vi "Userevent.vi"(0 "Timeout IN":i32, 7 "Source # startdelayLUT_coMD.vi?":bool, 9 "Source VI":string, 11 "Variable name":string, 12 "VI Match":bool, 13 "Value":variant) -> (4 "Timeout OUT":i32, 15 "shutdown?":bool)   [LabVIEW 2017]
uses:
  Custom Controls/display palette control.ctl
  Plugins/Macro Module/Macro Rule/subVIs/MacroRules_FGV_Commands.ctl
  CommonResource VIs/Timing/Timer Commands.ctl
  Custom Controls/pixel resolution enum.ctl
  Custom Controls/scan mode main settings tab.ctl
  Custom Controls/speed mode type def.ctl
  Custom Controls/experiment type.ctl
  Custom Controls/advanced settings inner tab CTL.ctl
  Custom Controls/MAIN Image panel tab Control type def.ctl
  Custom Controls/Histogram tab.ctl
  Custom Controls/trigger enum.ctl
  GFG/GFGDisplayRefsGet.vi
  GFG/GFGnumericGet.vi
  GFG/GFGfpRefGet.vi
  GFG/GFGbooleanGet.vi
  GFG/GFGImageRefsGet.vi
  GFG/GFG library.lvlib
panel:
  out "error out 6":errorcluster
  out "error out 5":errorcluster
  out "error out 4":errorcluster
  out "error out 3":errorcluster
  out "number of replacements":i32
  out "error out 2":errorcluster
  out "Source VI 2":string
  in  "String":string
  out "Maximum time delay observed":u32
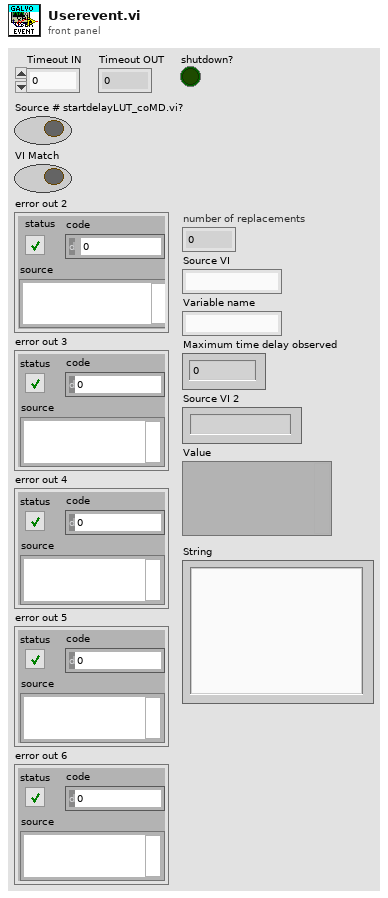
[diagram p1: front panel]
types:
  T1 = typedef "display palette control.ctl" = enum16{"standard", "high clipping red", "low clipping blue", "high and low clipping", "high / low (full range)"}
  T2 = typedef "MacroRules_FGV_Commands.ctl" = enum16{"Read File", "Get All", "Get Param and Flags"}
  T3 = typedef "Timer Commands.ctl" = enum16{"Clear All", "Start", "Pause", "Check Time"}
  T4 = enum8{"Enabled", "Disabled", "Disabled and Grayed Out"}
  T5 = typedef "pixel resolution enum.ctl" = enum16{"128 x 128", "256 x 128", "256 x 256", "512 x  64", "512 x 128", "512 x 256", "512 x 512", "1024 x 512", "1024 x 1024", "arbitrary"}
  T6 = typedef "scan mode main settings tab.ctl" = enum32{"2D frame", "2D line scan", "general settings", "Z Stack", "piezo"}
  T7 = typedef "experiment type.ctl" = string
  T8 = cluster{"xyvoltagefor2frames":dbl[][][], "x.pixels":dbl, "nomin.x.pixels":dbl, "y.pixels":dbl, "fill.fraction":dbl, "x.bidirectional":bool, "y.bidirectional":bool}
  T9 = enum32{"Page Enabled", "Page Disabled", "Page Disabled & Grayed"}
  T10 = typedef "advanced settings inner tab CTL.ctl" = enum32{"arb. frames", "AO", "AI", "channels", "trigger", "Zstack data"}
  T11 = typedef "MAIN Image panel tab Control type def.ctl" = enum32{"Channel 1", "Channel 2", "Channel 3", "Channel 4", "all channels", "RGB overlay", "ROI", "arbitrary line scan"}
  T12 = typedef "Histogram tab.ctl" = enum32{"hist Ch 1", "hist Ch 4", "hist Ch 3", "hist Ch 2"}
  T13 = typedef "trigger enum.ctl" = enum16{"legacy frame pulser PFI4", "continuous pulses", "single pulse", "trigger off"}
  T14 = cluster{"Channel 1 small":refnum<vi>, "Channel 2 small":refnum<vi>, "Channel 3 small":refnum<vi>, "Channel 4 small":refnum<vi>, "Channel 1 large":refnum<vi>, "Channel 2 large":refnum<vi>, "Channel 3 large":refnum<vi>, "Channel 4 large":refnum<vi>, "RGB overlay":refnum<vi>, "ROI Image display":refnum<vi>, "arb line scan display":refnum<vi>, "Channel 5 large":refnum<vi>}
  T15 = cluster{"WaveformChartRef":refnum<vi>, "DigitalRef":refnum<vi>, "ArrayRef":refnum<vi>, "TabControlRef":refnum<vi>, "EnumRef":refnum<vi>, "RingRef":refnum<vi>, "BooleanRef":refnum<vi>, "KnobRef":refnum<vi>, "SlideRef":refnum<vi>, "PathRef":refnum<vi>, "StringRef":refnum<vi>, "ComboBox":refnum<vi>, "WaveformGraphRef":refnum<vi>}
  T16 = typedef "IMAQ Image.ctl" = refnum<image>
  T17 = cluster{"Channel 1 small":T16, "Channel 2 small":T16, "Channel 3 small":T16, "Channel 4 small":T16, "Channel 1 large":T16, "Channel 2 large":T16, "Channel 3 large":T16, "Channel 4 large":T16, "RGB overlay":T16, "ROI Image display":T16, "arb line scan display":T16, "Channel 5 large":T16}
  T18 = typedef "speed mode type def.ctl" = u16
  T19 = typedef "LVStringsAndValuesArrayTypeDef.ctl" = cluster{"String":string, "Value":ext}[]
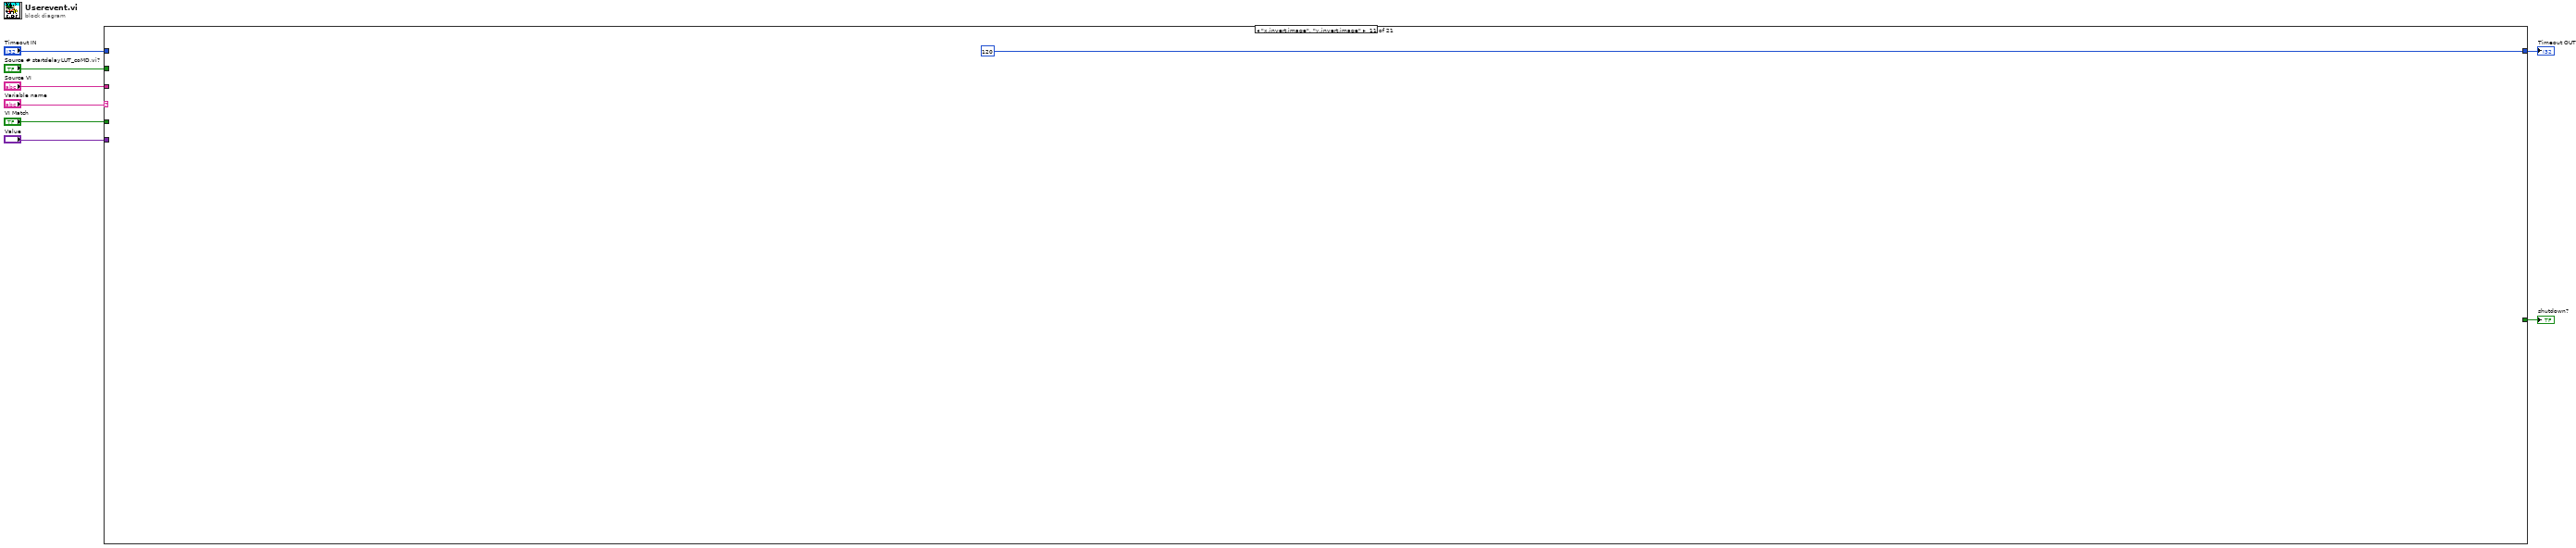
[diagram p0: block diagram]
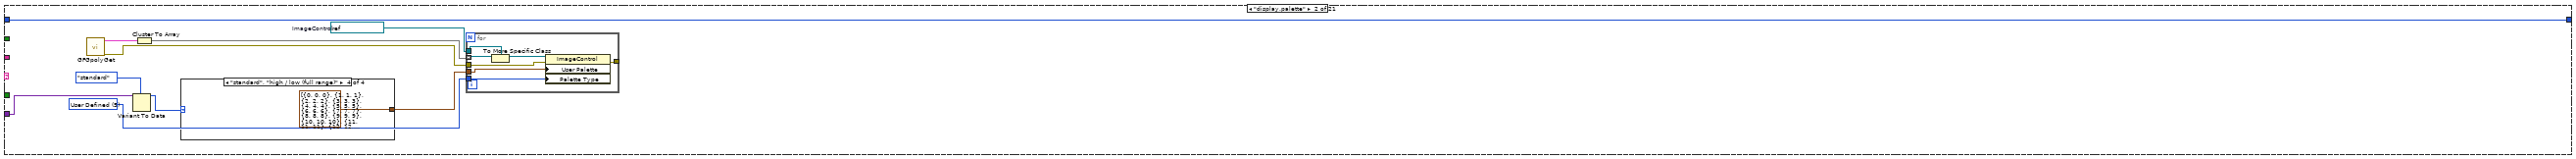
[diagram p3: hidden frame]
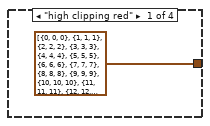
[diagram p4: hidden frame]
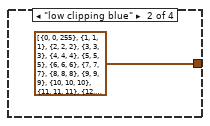
[diagram p5: hidden frame]
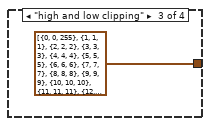
[diagram p6: hidden frame]
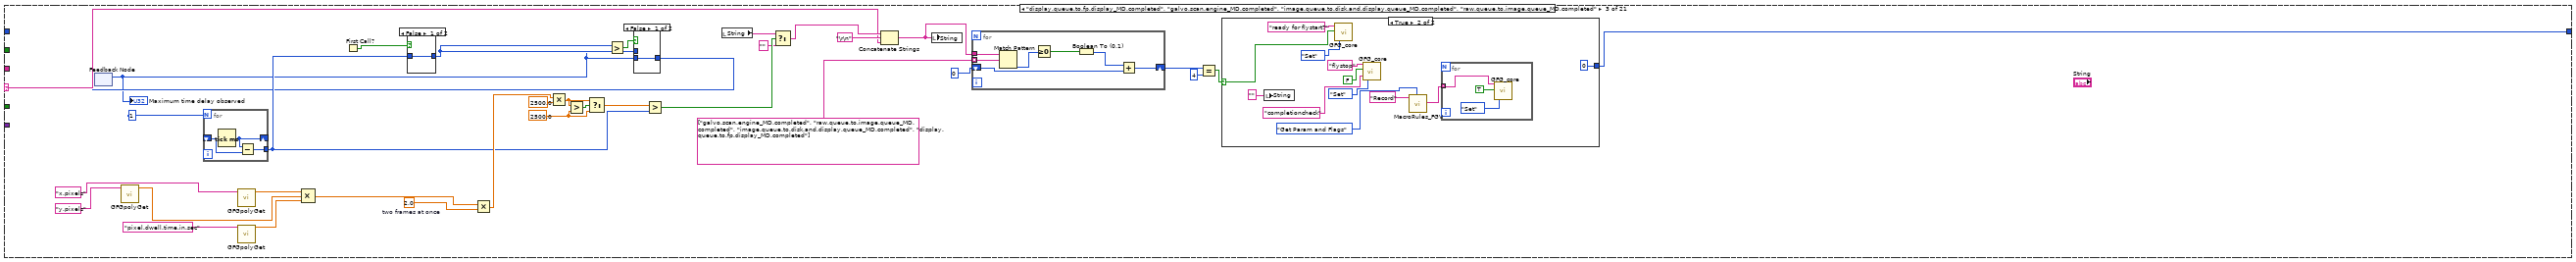
[diagram p7: hidden frame]
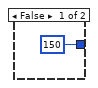
[diagram p8: hidden frame]
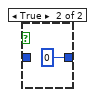
[diagram p9: hidden frame]
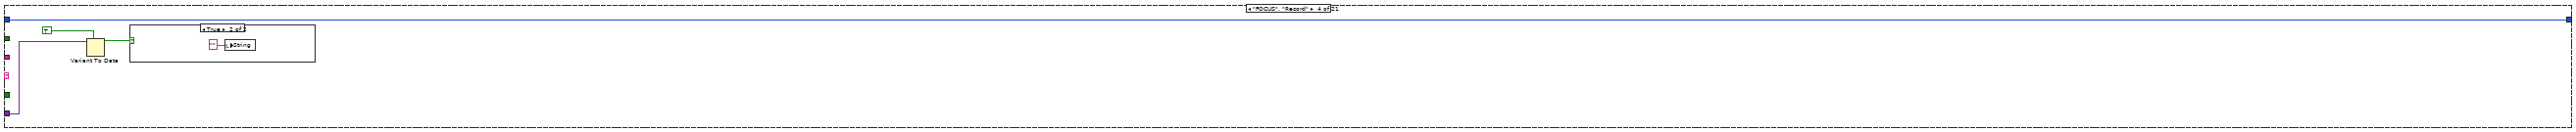
[diagram p11: hidden frame]
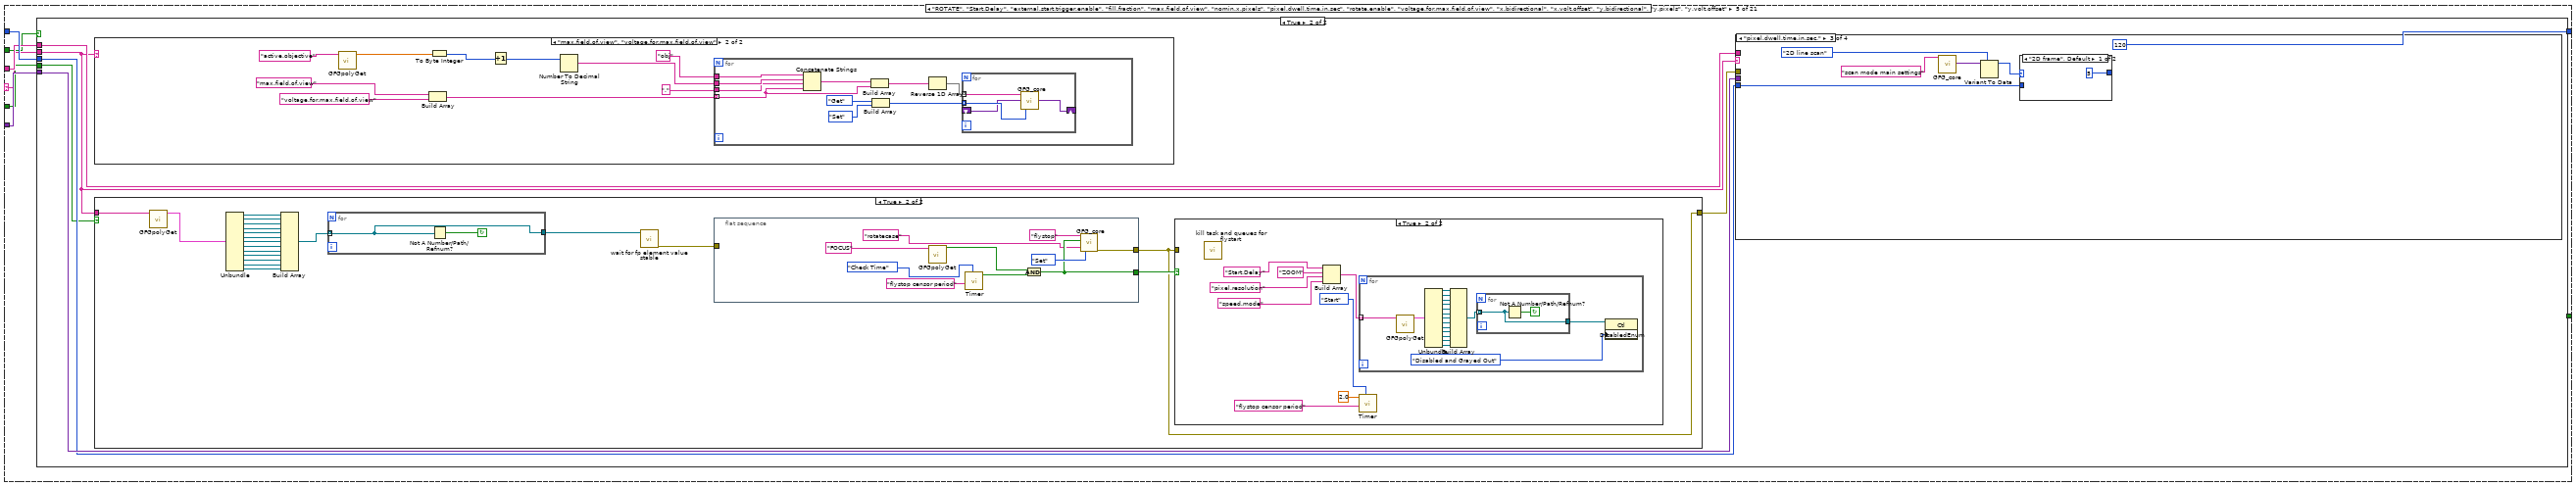
[diagram p13: hidden frame]
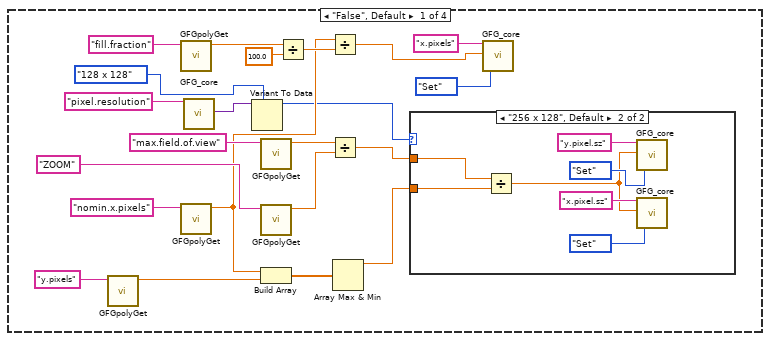
[diagram p18: hidden frame]
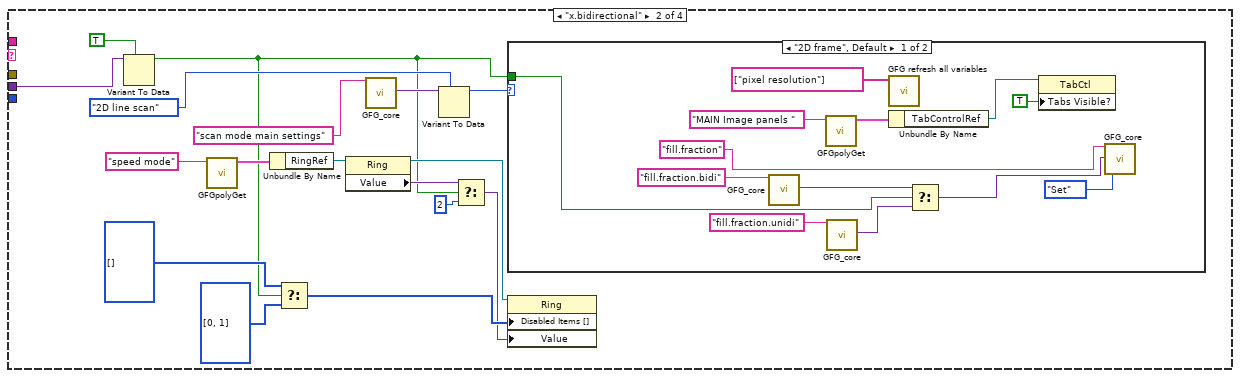
[diagram p20: hidden frame]
diagram:
  n1 = case shown="\"x.invert.image\", \"y.invert.image\"" "Variable name" {
    selector: "Variable name" -> [_ _ w54 _ w101 _ _ w311 _ w349 _ _ w620 _ _ _ _ _ _ _ _]
    tunnel: [_ _ _ _ _ _ _ _ _ _ _ _ _ _ _ _ _ _ TRUE _ _] -> w1
    tunnel: "Value" -> [_ w14 _ w98 w106 _ w289 _ _ w347 _ w601 w619 _ w712 w817 w872 w899 _ w953 w981]
    tunnel: [w9 w10 w53 w95 120 20 w302 w312 w338 w355 120 ("Timeout IN") w602 w618 w667 w708 w814 w871 w900 w919 w948 w975] -> w2
    tunnel: "Timeout IN" -> [w9 w10 _ w95 w105 _ w302 w312 w338 w344 _ w602 w618 w667 w709 w815 w871 w900 w919 w948 w975]
    tunnel: "Source VI" -> [_ _ _ _ w104 _ _ _ _ w353 _ _ _ w663 _ _ _ _ _ _ _]
    tunnel: "VI Match" -> [_ _ _ _ w102 _ _ _ _ w354 _ _ _ _ _ _ _ _ _ _ _]
    tunnel: "Source # startdelayLUT_coMD.vi?" -> [_ _ _ _ w100 _ _ _ _ _ _ _ _ _ _ _ _ _ _ _ _]
    frame "False", Default {
    }
    frame "display.palette" {
      w15 = u32 5 items=["Grayscale", "Binary", "Gradient", "Rainbow", "Temperature", "User Defined"] ("Palette:Palette Type")
      w17 = refnum<vi> refnum  # ImageControl
      n2 = call-poly "GFGpolyGet.vi"() -> ("error out"=w19:errorcluster, "DisplayRefsOut(generic class)"=w18:T14)  [unwired: 10 in]
      n3 = Variant To Data(type=display_palette_control."standard" ("display palette"), Variant=w14) -> (data=w12:T1)  [unwired: 1 in, 1 out]
      n4 = Cluster To Array(cluster=w18) -> (array=w16:refnum<vi>[])
      n5 = case shown="\"standard\", \"high / low (full range)\"" w12 {
        tunnel: [cluster{"Red":u8, "Green":u8, "Blue":u8}[] [{"Red"=0, "Green"=0, "Blue"=0}, {"Red"=1, "Green"=1, "Blue"=1}, {"Red"=2, "Green"=2, "Blue"=2}, {"Red"=3, "Green"=3, "Blue"=3}, {"Red"=4, "Green"=4, "Blue"=4}, {"Red"=5, "Green"=5, "Blue"=5}, {"Red"=6, "Green"=6, "Blue"=6}, {"Red"=7, "Green"=7, "Blue"=7}, {"Red"=8, "Green"=8, "Blue"=8}, {"Red"=9, "Green"=9, "Blue"=9}, {"Red"=10, "Green"=10, "Blue"=10}, {"Red"=11, "Green"=11, "Blue"=11}, {"Red"=12, "Green"=12, "Blue"=12}, {"Red"=13, "Green"=13, "Blue"=13}, {"Red"=14, "Green"=14, "Blue"=14}, {"Red"=15, "Green"=15, "Blue"=15}, {"Red"=16, "Green"=16, "Blue"=16}, {"Red"=17, "Green"=17, "Blue"=17}, {"Red"=18, "Green"=18, "Blue"=18}, {"Red"=19, "Green"=19, "Blue"=19}, {"Red"=20, "Green"=20, "Blue"=20}, {"Red"=21, "Green"=21, "Blue"=21}, {"Red"=22, "Green"=22, "Blue"=22}, {"Red"=23, "Green"=23, "Blue"=23}, {"Red"=24, "Green"=24, "Blue"=24}, {"Red"=25, "Green"=25, "Blue"=25}, {"Red"=26, "Green"=26, "Blue"=26}, {"Red"=27, "Green"=27, "Blue"=27}, {"Red"=28, "Green"=28, "Blue"=28}, {"Red"=29, "Green"=29, "Blue"=29}, {"Red"=30, "Green"=30, "Blue"=30}, {"Red"=31, "Green"=31, "Blue"=31}, {"Red"=32, "Green"=32, "Blue"=32}, {"Red"=33, "Green"=33, "Blue"=33}, {"Red"=34, "Green"=34, "Blue"=34}, {"Red"=35, "Green"=35, "Blue"=35}, {"Red"=36, "Green"=36, "Blue"=36}, {"Red"=37, "Green"=37, "Blue"=37}, {"Red"=38, "Green"=38, "Blue"=38}, {"Red"=39, "Green"=39, "Blue"=39}, {"Red"=40, "Green"=40, "Blue"=40}, {"Red"=41, "Green"=41, "Blue"=41}, {"Red"=42, "Green"=42, "Blue"=42}, {"Red"=43, "Green"=43, "Blue"=43}, {"Red"=44, "Green"=44, "Blue"=44}, {"Red"=45, "Green"=45, "Blue"=45}, {"Red"=46, "Green"=46, "Blue"=46}, {"Red"=47, "Green"=47, "Blue"=47}, {"Red"=48, "Green"=48, "Blue"=48}, {"Red"=49, "Green"=49, "Blue"=49}, {"Red"=50, "Green"=50, "Blue"=50}, {"Red"=51, "Green"=51, "Blue"=51}, {"Red"=52, "Green"=52, "Blue"=52}, {"Red"=53, "Green"=53, "Blue"=53}, {"Red"=54, "Green"=54, "Blue"=54}, {"Red"=55, "Green"=55, "Blue"=55}, {"Red"=56, "Green"=56, "Blue"=56}, {"Red"=57, "Green"=57, "Blue"=57}, {"Red"=58, "Green"=58, "Blue"=58}, {"Red"=59, "Green"=59, "Blue"=59}, {"Red"=60, "Green"=60, "Blue"=60}, {"Red"=61, "Green"=61, "Blue"=61}, {"Red"=62, "Green"=62, "Blue"=62}, {"Red"=63, "Green"=63, "Blue"=63}, {"Red"=64, "Green"=64, "Blue"=64}, {"Red"=65, "Green"=65, "Blue"=65}, {"Red"=66, "Green"=66, "Blue"=66}, {"Red"=67, "Green"=67, "Blue"=67}, {"Red"=68, "Green"=68, "Blue"=68}, {"Red"=69, "Green"=69, "Blue"=69}, {"Red"=70, "Green"=70, "Blue"=70}, {"Red"=71, "Green"=71, "Blue"=71}, {"Red"=72, "Green"=72, "Blue"=72}, {"Red"=73, "Green"=73, "Blue"=73}, {"Red"=74, "Green"=74, "Blue"=74}, {"Red"=75, "Green"=75, "Blue"=75}, {"Red"=76, "Green"=76, "Blue"=76}, {"Red"=77, "Green"=77, "Blue"=77}, {"Red"=78, "Green"=78, "Blue"=78}, {"Red"=79, "Green"=79, "Blue"=79}, {"Red"=80, "Green"=80, "Blue"=80}, {"Red"=81, "Green"=81, "Blue"=81}, {"Red"=82, "Green"=82, "Blue"=82}, {"Red"=83, "Green"=83, "Blue"=83}, {"Red"=84, "Green"=84, "Blue"=84}, {"Red"=85, "Green"=85, "Blue"=85}, {"Red"=86, "Green"=86, "Blue"=86}, {"Red"=87, "Green"=87, "Blue"=87}, {"Red"=88, "Green"=88, "Blue"=88}, {"Red"=89, "Green"=89, "Blue"=89}, {"Red"=90, "Green"=90, "Blue"=90}, {"Red"=91, "Green"=91, "Blue"=91}, {"Red"=92, "Green"=92, "Blue"=92}, {"Red"=93, "Green"=93, "Blue"=93}, {"Red"=94, "Green"=94, "Blue"=94}, {"Red"=95, "Green"=95, "Blue"=95}, {"Red"=96, "Green"=96, "Blue"=96}, {"Red"=97, "Green"=97, "Blue"=97}, {"Red"=98, "Green"=98, "Blue"=98}, {"Red"=99, "Green"=99, "Blue"=99}, {"Red"=100, "Green"=100, "Blue"=100}, {"Red"=101, "Green"=101, "Blue"=101}, {"Red"=102, "Green"=102, "Blue"=102}, {"Red"=103, "Green"=103, "Blue"=103}, {"Red"=104, "Green"=104, "Blue"=104}, {"Red"=105, "Green"=105, "Blue"=105}, {"Red"=106, "Green"=106, "Blue"=106}, {"Red"=107, "Green"=107, "Blue"=107}, {"Red"=108, "Green"=108, "Blue"=108}, {"Red"=109, "Green"=109, "Blue"=109}, {"Red"=110, "Green"=110, "Blue"=110}, {"Red"=111, "Green"=111, "Blue"=111}, {"Red"=112, "Green"=112, "Blue"=112}, {"Red"=113, "Green"=113, "Blue"=113}, {"Red"=114, "Green"=114, "Blue"=114}, {"Red"=115, "Green"=115, "Blue"=115}, {"Red"=116, "Green"=116, "Blue"=116}, {"Red"=117, "Green"=117, "Blue"=117}, {"Red"=118, "Green"=118, "Blue"=118}, {"Red"=119, "Green"=119, "Blue"=119}, {"Red"=120, "Green"=120, "Blue"=120}, {"Red"=121, "Green"=121, "Blue"=121}, {"Red"=122, "Green"=122, "Blue"=122}, {"Red"=123, "Green"=123, "Blue"=123}, {"Red"=124, "Green"=124, "Blue"=124}, {"Red"=125, "Green"=125, "Blue"=125}, {"Red"=126, "Green"=126, "Blue"=126}, {"Red"=127, "Green"=127, "Blue"=127}, {"Red"=128, "Green"=128, "Blue"=128}, {"Red"=129, "Green"=129, "Blue"=129}, {"Red"=130, "Green"=130, "Blue"=130}, {"Red"=131, "Green"=131, "Blue"=131}, {"Red"=132, "Green"=132, "Blue"=132}, {"Red"=133, "Green"=133, "Blue"=133}, {"Red"=134, "Green"=134, "Blue"=134}, {"Red"=135, "Green"=135, "Blue"=135}, {"Red"=136, "Green"=136, "Blue"=136}, {"Red"=137, "Green"=137, "Blue"=137}, {"Red"=138, "Green"=138, "Blue"=138}, {"Red"=139, "Green"=139, "Blue"=139}, {"Red"=140, "Green"=140, "Blue"=140}, {"Red"=141, "Green"=141, "Blue"=141}, {"Red"=142, "Green"=142, "Blue"=142}, {"Red"=143, "Green"=143, "Blue"=143}, {"Red"=144, "Green"=144, "Blue"=144}, {"Red"=145, "Green"=145, "Blue"=145}, {"Red"=146, "Green"=146, "Blue"=146}, {"Red"=147, "Green"=147, "Blue"=147}, {"Red"=148, "Green"=148, "Blue"=148}, {"Red"=149, "Green"=149, "Blue"=149}, {"Red"=150, "Green"=150, "Blue"=150}, {"Red"=151, "Green"=151, "Blue"=151}, {"Red"=152, "Green"=152, "Blue"=152}, {"Red"=153, "Green"=153, "Blue"=153}, {"Red"=154, "Green"=154, "Blue"=154}, {"Red"=155, "Green"=155, "Blue"=155}, {"Red"=156, "Green"=156, "Blue"=156}, {"Red"=157, "Green"=157, "Blue"=157}, {"Red"=158, "Green"=158, "Blue"=158}, {"Red"=159, "Green"=159, "Blue"=159}, {"Red"=160, "Green"=160, "Blue"=160}, {"Red"=161, "Green"=161, "Blue"=161}, {"Red"=162, "Green"=162, "Blue"=162}, {"Red"=163, "Green"=163, "Blue"=163}, {"Red"=164, "Green"=164, "Blue"=164}, {"Red"=165, "Green"=165, "Blue"=165}, {"Red"=166, "Green"=166, "Blue"=166}, {"Red"=167, "Green"=167, "Blue"=167}, {"Red"=168, "Green"=168, "Blue"=168}, {"Red"=169, "Green"=169, "Blue"=169}, {"Red"=170, "Green"=170, "Blue"=170}, {"Red"=171, "Green"=171, "Blue"=171}, {"Red"=172, "Green"=172, "Blue"=172}, {"Red"=173, "Green"=173, "Blue"=173}, {"Red"=174, "Green"=174, "Blue"=174}, {"Red"=175, "Green"=175, "Blue"=175}, {"Red"=176, "Green"=176, "Blue"=176}, {"Red"=177, "Green"=177, "Blue"=177}, {"Red"=178, "Green"=178, "Blue"=178}, {"Red"=179, "Green"=179, "Blue"=179}, {"Red"=180, "Green"=180, "Blue"=180}, {"Red"=181, "Green"=181, "Blue"=181}, {"Red"=182, "Green"=182, "Blue"=182}, {"Red"=183, "Green"=183, "Blue"=183}, {"Red"=184, "Green"=184, "Blue"=184}, {"Red"=185, "Green"=185, "Blue"=185}, {"Red"=186, "Green"=186, "Blue"=186}, {"Red"=187, "Green"=187, "Blue"=187}, {"Red"=188, "Green"=188, "Blue"=188}, {"Red"=189, "Green"=189, "Blue"=189}, {"Red"=190, "Green"=190, "Blue"=190}, {"Red"=191, "Green"=191, "Blue"=191}, {"Red"=192, "Green"=192, "Blue"=192}, {"Red"=193, "Green"=193, "Blue"=193}, {"Red"=194, "Green"=194, "Blue"=194}, {"Red"=195, "Green"=195, "Blue"=195}, {"Red"=196, "Green"=196, "Blue"=196}, {"Red"=197, "Green"=197, "Blue"=197}, {"Red"=198, "Green"=198, "Blue"=198}, {"Red"=199, "Green"=199, "Blue"=199}, {"Red"=200, "Green"=200, "Blue"=200}, {"Red"=201, "Green"=201, "Blue"=201}, {"Red"=202, "Green"=202, "Blue"=202}, {"Red"=203, "Green"=203, "Blue"=203}, {"Red"=204, "Green"=204, "Blue"=204}, {"Red"=205, "Green"=205, "Blue"=205}, {"Red"=206, "Green"=206, "Blue"=206}, {"Red"=207, "Green"=207, "Blue"=207}, {"Red"=208, "Green"=208, "Blue"=208}, {"Red"=209, "Green"=209, "Blue"=209}, {"Red"=210, "Green"=210, "Blue"=210}, {"Red"=211, "Green"=211, "Blue"=211}, {"Red"=212, "Green"=212, "Blue"=212}, {"Red"=213, "Green"=213, "Blue"=213}, {"Red"=214, "Green"=214, "Blue"=214}, {"Red"=215, "Green"=215, "Blue"=215}, {"Red"=216, "Green"=216, "Blue"=216}, {"Red"=217, "Green"=217, "Blue"=217}, {"Red"=218, "Green"=218, "Blue"=218}, {"Red"=219, "Green"=219, "Blue"=219}, {"Red"=220, "Green"=220, "Blue"=220}, {"Red"=221, "Green"=221, "Blue"=221}, {"Red"=222, "Green"=222, "Blue"=222}, {"Red"=223, "Green"=223, "Blue"=223}, {"Red"=224, "Green"=224, "Blue"=224}, {"Red"=225, "Green"=225, "Blue"=225}, {"Red"=226, "Green"=226, "Blue"=226}, {"Red"=227, "Green"=227, "Blue"=227}, {"Red"=228, "Green"=228, "Blue"=228}, {"Red"=229, "Green"=229, "Blue"=229}, {"Red"=230, "Green"=230, "Blue"=230}, {"Red"=231, "Green"=231, "Blue"=231}, {"Red"=232, "Green"=232, "Blue"=232}, {"Red"=233, "Green"=233, "Blue"=233}, {"Red"=234, "Green"=234, "Blue"=234}, {"Red"=235, "Green"=235, "Blue"=235}, {"Red"=236, "Green"=236, "Blue"=236}, {"Red"=237, "Green"=237, "Blue"=237}, {"Red"=238, "Green"=238, "Blue"=238}, {"Red"=239, "Green"=239, "Blue"=239}, {"Red"=240, "Green"=240, "Blue"=240}, {"Red"=241, "Green"=241, "Blue"=241}, {"Red"=242, "Green"=242, "Blue"=242}, {"Red"=243, "Green"=243, "Blue"=243}, {"Red"=244, "Green"=244, "Blue"=244}, {"Red"=245, "Green"=245, "Blue"=245}, {"Red"=246, "Green"=246, "Blue"=246}, {"Red"=247, "Green"=247, "Blue"=247}, {"Red"=248, "Green"=248, "Blue"=248}, {"Red"=249, "Green"=249, "Blue"=249}, {"Red"=250, "Green"=250, "Blue"=250}, {"Red"=251, "Green"=251, "Blue"=251}, {"Red"=252, "Green"=252, "Blue"=252}, {"Red"=253, "Green"=253, "Blue"=253}, {"Red"=254, "Green"=254, "Blue"=254}, {"Red"=255, "Green"=0, "Blue"=0}] ("Color Palette") cluster{"Red":u8, "Green":u8, "Blue":u8}[] [{"Red"=0, "Green"=0, "Blue"=255}, {"Red"=1, "Green"=1, "Blue"=1}, {"Red"=2, "Green"=2, "Blue"=2}, {"Red"=3, "Green"=3, "Blue"=3}, {"Red"=4, "Green"=4, "Blue"=4}, {"Red"=5, "Green"=5, "Blue"=5}, {"Red"=6, "Green"=6, "Blue"=6}, {"Red"=7, "Green"=7, "Blue"=7}, {"Red"=8, "Green"=8, "Blue"=8}, {"Red"=9, "Green"=9, "Blue"=9}, {"Red"=10, "Green"=10, "Blue"=10}, {"Red"=11, "Green"=11, "Blue"=11}, {"Red"=12, "Green"=12, "Blue"=12}, {"Red"=13, "Green"=13, "Blue"=13}, {"Red"=14, "Green"=14, "Blue"=14}, {"Red"=15, "Green"=15, "Blue"=15}, {"Red"=16, "Green"=16, "Blue"=16}, {"Red"=17, "Green"=17, "Blue"=17}, {"Red"=18, "Green"=18, "Blue"=18}, {"Red"=19, "Green"=19, "Blue"=19}, {"Red"=20, "Green"=20, "Blue"=20}, {"Red"=21, "Green"=21, "Blue"=21}, {"Red"=22, "Green"=22, "Blue"=22}, {"Red"=23, "Green"=23, "Blue"=23}, {"Red"=24, "Green"=24, "Blue"=24}, {"Red"=25, "Green"=25, "Blue"=25}, {"Red"=26, "Green"=26, "Blue"=26}, {"Red"=27, "Green"=27, "Blue"=27}, {"Red"=28, "Green"=28, "Blue"=28}, {"Red"=29, "Green"=29, "Blue"=29}, {"Red"=30, "Green"=30, "Blue"=30}, {"Red"=31, "Green"=31, "Blue"=31}, {"Red"=32, "Green"=32, "Blue"=32}, {"Red"=33, "Green"=33, "Blue"=33}, {"Red"=34, "Green"=34, "Blue"=34}, {"Red"=35, "Green"=35, "Blue"=35}, {"Red"=36, "Green"=36, "Blue"=36}, {"Red"=37, "Green"=37, "Blue"=37}, {"Red"=38, "Green"=38, "Blue"=38}, {"Red"=39, "Green"=39, "Blue"=39}, {"Red"=40, "Green"=40, "Blue"=40}, {"Red"=41, "Green"=41, "Blue"=41}, {"Red"=42, "Green"=42, "Blue"=42}, {"Red"=43, "Green"=43, "Blue"=43}, {"Red"=44, "Green"=44, "Blue"=44}, {"Red"=45, "Green"=45, "Blue"=45}, {"Red"=46, "Green"=46, "Blue"=46}, {"Red"=47, "Green"=47, "Blue"=47}, {"Red"=48, "Green"=48, "Blue"=48}, {"Red"=49, "Green"=49, "Blue"=49}, {"Red"=50, "Green"=50, "Blue"=50}, {"Red"=51, "Green"=51, "Blue"=51}, {"Red"=52, "Green"=52, "Blue"=52}, {"Red"=53, "Green"=53, "Blue"=53}, {"Red"=54, "Green"=54, "Blue"=54}, {"Red"=55, "Green"=55, "Blue"=55}, {"Red"=56, "Green"=56, "Blue"=56}, {"Red"=57, "Green"=57, "Blue"=57}, {"Red"=58, "Green"=58, "Blue"=58}, {"Red"=59, "Green"=59, "Blue"=59}, {"Red"=60, "Green"=60, "Blue"=60}, {"Red"=61, "Green"=61, "Blue"=61}, {"Red"=62, "Green"=62, "Blue"=62}, {"Red"=63, "Green"=63, "Blue"=63}, {"Red"=64, "Green"=64, "Blue"=64}, {"Red"=65, "Green"=65, "Blue"=65}, {"Red"=66, "Green"=66, "Blue"=66}, {"Red"=67, "Green"=67, "Blue"=67}, {"Red"=68, "Green"=68, "Blue"=68}, {"Red"=69, "Green"=69, "Blue"=69}, {"Red"=70, "Green"=70, "Blue"=70}, {"Red"=71, "Green"=71, "Blue"=71}, {"Red"=72, "Green"=72, "Blue"=72}, {"Red"=73, "Green"=73, "Blue"=73}, {"Red"=74, "Green"=74, "Blue"=74}, {"Red"=75, "Green"=75, "Blue"=75}, {"Red"=76, "Green"=76, "Blue"=76}, {"Red"=77, "Green"=77, "Blue"=77}, {"Red"=78, "Green"=78, "Blue"=78}, {"Red"=79, "Green"=79, "Blue"=79}, {"Red"=80, "Green"=80, "Blue"=80}, {"Red"=81, "Green"=81, "Blue"=81}, {"Red"=82, "Green"=82, "Blue"=82}, {"Red"=83, "Green"=83, "Blue"=83}, {"Red"=84, "Green"=84, "Blue"=84}, {"Red"=85, "Green"=85, "Blue"=85}, {"Red"=86, "Green"=86, "Blue"=86}, {"Red"=87, "Green"=87, "Blue"=87}, {"Red"=88, "Green"=88, "Blue"=88}, {"Red"=89, "Green"=89, "Blue"=89}, {"Red"=90, "Green"=90, "Blue"=90}, {"Red"=91, "Green"=91, "Blue"=91}, {"Red"=92, "Green"=92, "Blue"=92}, {"Red"=93, "Green"=93, "Blue"=93}, {"Red"=94, "Green"=94, "Blue"=94}, {"Red"=95, "Green"=95, "Blue"=95}, {"Red"=96, "Green"=96, "Blue"=96}, {"Red"=97, "Green"=97, "Blue"=97}, {"Red"=98, "Green"=98, "Blue"=98}, {"Red"=99, "Green"=99, "Blue"=99}, {"Red"=100, "Green"=100, "Blue"=100}, {"Red"=101, "Green"=101, "Blue"=101}, {"Red"=102, "Green"=102, "Blue"=102}, {"Red"=103, "Green"=103, "Blue"=103}, {"Red"=104, "Green"=104, "Blue"=104}, {"Red"=105, "Green"=105, "Blue"=105}, {"Red"=106, "Green"=106, "Blue"=106}, {"Red"=107, "Green"=107, "Blue"=107}, {"Red"=108, "Green"=108, "Blue"=108}, {"Red"=109, "Green"=109, "Blue"=109}, {"Red"=110, "Green"=110, "Blue"=110}, {"Red"=111, "Green"=111, "Blue"=111}, {"Red"=112, "Green"=112, "Blue"=112}, {"Red"=113, "Green"=113, "Blue"=113}, {"Red"=114, "Green"=114, "Blue"=114}, {"Red"=115, "Green"=115, "Blue"=115}, {"Red"=116, "Green"=116, "Blue"=116}, {"Red"=117, "Green"=117, "Blue"=117}, {"Red"=118, "Green"=118, "Blue"=118}, {"Red"=119, "Green"=119, "Blue"=119}, {"Red"=120, "Green"=120, "Blue"=120}, {"Red"=121, "Green"=121, "Blue"=121}, {"Red"=122, "Green"=122, "Blue"=122}, {"Red"=123, "Green"=123, "Blue"=123}, {"Red"=124, "Green"=124, "Blue"=124}, {"Red"=125, "Green"=125, "Blue"=125}, {"Red"=126, "Green"=126, "Blue"=126}, {"Red"=127, "Green"=127, "Blue"=127}, {"Red"=128, "Green"=128, "Blue"=128}, {"Red"=129, "Green"=129, "Blue"=129}, {"Red"=130, "Green"=130, "Blue"=130}, {"Red"=131, "Green"=131, "Blue"=131}, {"Red"=132, "Green"=132, "Blue"=132}, {"Red"=133, "Green"=133, "Blue"=133}, {"Red"=134, "Green"=134, "Blue"=134}, {"Red"=135, "Green"=135, "Blue"=135}, {"Red"=136, "Green"=136, "Blue"=136}, {"Red"=137, "Green"=137, "Blue"=137}, {"Red"=138, "Green"=138, "Blue"=138}, {"Red"=139, "Green"=139, "Blue"=139}, {"Red"=140, "Green"=140, "Blue"=140}, {"Red"=141, "Green"=141, "Blue"=141}, {"Red"=142, "Green"=142, "Blue"=142}, {"Red"=143, "Green"=143, "Blue"=143}, {"Red"=144, "Green"=144, "Blue"=144}, {"Red"=145, "Green"=145, "Blue"=145}, {"Red"=146, "Green"=146, "Blue"=146}, {"Red"=147, "Green"=147, "Blue"=147}, {"Red"=148, "Green"=148, "Blue"=148}, {"Red"=149, "Green"=149, "Blue"=149}, {"Red"=150, "Green"=150, "Blue"=150}, {"Red"=151, "Green"=151, "Blue"=151}, {"Red"=152, "Green"=152, "Blue"=152}, {"Red"=153, "Green"=153, "Blue"=153}, {"Red"=154, "Green"=154, "Blue"=154}, {"Red"=155, "Green"=155, "Blue"=155}, {"Red"=156, "Green"=156, "Blue"=156}, {"Red"=157, "Green"=157, "Blue"=157}, {"Red"=158, "Green"=158, "Blue"=158}, {"Red"=159, "Green"=159, "Blue"=159}, {"Red"=160, "Green"=160, "Blue"=160}, {"Red"=161, "Green"=161, "Blue"=161}, {"Red"=162, "Green"=162, "Blue"=162}, {"Red"=163, "Green"=163, "Blue"=163}, {"Red"=164, "Green"=164, "Blue"=164}, {"Red"=165, "Green"=165, "Blue"=165}, {"Red"=166, "Green"=166, "Blue"=166}, {"Red"=167, "Green"=167, "Blue"=167}, {"Red"=168, "Green"=168, "Blue"=168}, {"Red"=169, "Green"=169, "Blue"=169}, {"Red"=170, "Green"=170, "Blue"=170}, {"Red"=171, "Green"=171, "Blue"=171}, {"Red"=172, "Green"=172, "Blue"=172}, {"Red"=173, "Green"=173, "Blue"=173}, {"Red"=174, "Green"=174, "Blue"=174}, {"Red"=175, "Green"=175, "Blue"=175}, {"Red"=176, "Green"=176, "Blue"=176}, {"Red"=177, "Green"=177, "Blue"=177}, {"Red"=178, "Green"=178, "Blue"=178}, {"Red"=179, "Green"=179, "Blue"=179}, {"Red"=180, "Green"=180, "Blue"=180}, {"Red"=181, "Green"=181, "Blue"=181}, {"Red"=182, "Green"=182, "Blue"=182}, {"Red"=183, "Green"=183, "Blue"=183}, {"Red"=184, "Green"=184, "Blue"=184}, {"Red"=185, "Green"=185, "Blue"=185}, {"Red"=186, "Green"=186, "Blue"=186}, {"Red"=187, "Green"=187, "Blue"=187}, {"Red"=188, "Green"=188, "Blue"=188}, {"Red"=189, "Green"=189, "Blue"=189}, {"Red"=190, "Green"=190, "Blue"=190}, {"Red"=191, "Green"=191, "Blue"=191}, {"Red"=192, "Green"=192, "Blue"=192}, {"Red"=193, "Green"=193, "Blue"=193}, {"Red"=194, "Green"=194, "Blue"=194}, {"Red"=195, "Green"=195, "Blue"=195}, {"Red"=196, "Green"=196, "Blue"=196}, {"Red"=197, "Green"=197, "Blue"=197}, {"Red"=198, "Green"=198, "Blue"=198}, {"Red"=199, "Green"=199, "Blue"=199}, {"Red"=200, "Green"=200, "Blue"=200}, {"Red"=201, "Green"=201, "Blue"=201}, {"Red"=202, "Green"=202, "Blue"=202}, {"Red"=203, "Green"=203, "Blue"=203}, {"Red"=204, "Green"=204, "Blue"=204}, {"Red"=205, "Green"=205, "Blue"=205}, {"Red"=206, "Green"=206, "Blue"=206}, {"Red"=207, "Green"=207, "Blue"=207}, {"Red"=208, "Green"=208, "Blue"=208}, {"Red"=209, "Green"=209, "Blue"=209}, {"Red"=210, "Green"=210, "Blue"=210}, {"Red"=211, "Green"=211, "Blue"=211}, {"Red"=212, "Green"=212, "Blue"=212}, {"Red"=213, "Green"=213, "Blue"=213}, {"Red"=214, "Green"=214, "Blue"=214}, {"Red"=215, "Green"=215, "Blue"=215}, {"Red"=216, "Green"=216, "Blue"=216}, {"Red"=217, "Green"=217, "Blue"=217}, {"Red"=218, "Green"=218, "Blue"=218}, {"Red"=219, "Green"=219, "Blue"=219}, {"Red"=220, "Green"=220, "Blue"=220}, {"Red"=221, "Green"=221, "Blue"=221}, {"Red"=222, "Green"=222, "Blue"=222}, {"Red"=223, "Green"=223, "Blue"=223}, {"Red"=224, "Green"=224, "Blue"=224}, {"Red"=225, "Green"=225, "Blue"=225}, {"Red"=226, "Green"=226, "Blue"=226}, {"Red"=227, "Green"=227, "Blue"=227}, {"Red"=228, "Green"=228, "Blue"=228}, {"Red"=229, "Green"=229, "Blue"=229}, {"Red"=230, "Green"=230, "Blue"=230}, {"Red"=231, "Green"=231, "Blue"=231}, {"Red"=232, "Green"=232, "Blue"=232}, {"Red"=233, "Green"=233, "Blue"=233}, {"Red"=234, "Green"=234, "Blue"=234}, {"Red"=235, "Green"=235, "Blue"=235}, {"Red"=236, "Green"=236, "Blue"=236}, {"Red"=237, "Green"=237, "Blue"=237}, {"Red"=238, "Green"=238, "Blue"=238}, {"Red"=239, "Green"=239, "Blue"=239}, {"Red"=240, "Green"=240, "Blue"=240}, {"Red"=241, "Green"=241, "Blue"=241}, {"Red"=242, "Green"=242, "Blue"=242}, {"Red"=243, "Green"=243, "Blue"=243}, {"Red"=244, "Green"=244, "Blue"=244}, {"Red"=245, "Green"=245, "Blue"=245}, {"Red"=246, "Green"=246, "Blue"=246}, {"Red"=247, "Green"=247, "Blue"=247}, {"Red"=248, "Green"=248, "Blue"=248}, {"Red"=249, "Green"=249, "Blue"=249}, {"Red"=250, "Green"=250, "Blue"=250}, {"Red"=251, "Green"=251, "Blue"=251}, {"Red"=252, "Green"=252, "Blue"=252}, {"Red"=253, "Green"=253, "Blue"=253}, {"Red"=254, "Green"=254, "Blue"=254}, {"Red"=255, "Green"=255, "Blue"=255}] ("Color Palette") cluster{"Red":u8, "Green":u8, "Blue":u8}[] [{"Red"=0, "Green"=0, "Blue"=255}, {"Red"=1, "Green"=1, "Blue"=1}, {"Red"=2, "Green"=2, "Blue"=2}, {"Red"=3, "Green"=3, "Blue"=3}, {"Red"=4, "Green"=4, "Blue"=4}, {"Red"=5, "Green"=5, "Blue"=5}, {"Red"=6, "Green"=6, "Blue"=6}, {"Red"=7, "Green"=7, "Blue"=7}, {"Red"=8, "Green"=8, "Blue"=8}, {"Red"=9, "Green"=9, "Blue"=9}, {"Red"=10, "Green"=10, "Blue"=10}, {"Red"=11, "Green"=11, "Blue"=11}, {"Red"=12, "Green"=12, "Blue"=12}, {"Red"=13, "Green"=13, "Blue"=13}, {"Red"=14, "Green"=14, "Blue"=14}, {"Red"=15, "Green"=15, "Blue"=15}, {"Red"=16, "Green"=16, "Blue"=16}, {"Red"=17, "Green"=17, "Blue"=17}, {"Red"=18, "Green"=18, "Blue"=18}, {"Red"=19, "Green"=19, "Blue"=19}, {"Red"=20, "Green"=20, "Blue"=20}, {"Red"=21, "Green"=21, "Blue"=21}, {"Red"=22, "Green"=22, "Blue"=22}, {"Red"=23, "Green"=23, "Blue"=23}, {"Red"=24, "Green"=24, "Blue"=24}, {"Red"=25, "Green"=25, "Blue"=25}, {"Red"=26, "Green"=26, "Blue"=26}, {"Red"=27, "Green"=27, "Blue"=27}, {"Red"=28, "Green"=28, "Blue"=28}, {"Red"=29, "Green"=29, "Blue"=29}, {"Red"=30, "Green"=30, "Blue"=30}, {"Red"=31, "Green"=31, "Blue"=31}, {"Red"=32, "Green"=32, "Blue"=32}, {"Red"=33, "Green"=33, "Blue"=33}, {"Red"=34, "Green"=34, "Blue"=34}, {"Red"=35, "Green"=35, "Blue"=35}, {"Red"=36, "Green"=36, "Blue"=36}, {"Red"=37, "Green"=37, "Blue"=37}, {"Red"=38, "Green"=38, "Blue"=38}, {"Red"=39, "Green"=39, "Blue"=39}, {"Red"=40, "Green"=40, "Blue"=40}, {"Red"=41, "Green"=41, "Blue"=41}, {"Red"=42, "Green"=42, "Blue"=42}, {"Red"=43, "Green"=43, "Blue"=43}, {"Red"=44, "Green"=44, "Blue"=44}, {"Red"=45, "Green"=45, "Blue"=45}, {"Red"=46, "Green"=46, "Blue"=46}, {"Red"=47, "Green"=47, "Blue"=47}, {"Red"=48, "Green"=48, "Blue"=48}, {"Red"=49, "Green"=49, "Blue"=49}, {"Red"=50, "Green"=50, "Blue"=50}, {"Red"=51, "Green"=51, "Blue"=51}, {"Red"=52, "Green"=52, "Blue"=52}, {"Red"=53, "Green"=53, "Blue"=53}, {"Red"=54, "Green"=54, "Blue"=54}, {"Red"=55, "Green"=55, "Blue"=55}, {"Red"=56, "Green"=56, "Blue"=56}, {"Red"=57, "Green"=57, "Blue"=57}, {"Red"=58, "Green"=58, "Blue"=58}, {"Red"=59, "Green"=59, "Blue"=59}, {"Red"=60, "Green"=60, "Blue"=60}, {"Red"=61, "Green"=61, "Blue"=61}, {"Red"=62, "Green"=62, "Blue"=62}, {"Red"=63, "Green"=63, "Blue"=63}, {"Red"=64, "Green"=64, "Blue"=64}, {"Red"=65, "Green"=65, "Blue"=65}, {"Red"=66, "Green"=66, "Blue"=66}, {"Red"=67, "Green"=67, "Blue"=67}, {"Red"=68, "Green"=68, "Blue"=68}, {"Red"=69, "Green"=69, "Blue"=69}, {"Red"=70, "Green"=70, "Blue"=70}, {"Red"=71, "Green"=71, "Blue"=71}, {"Red"=72, "Green"=72, "Blue"=72}, {"Red"=73, "Green"=73, "Blue"=73}, {"Red"=74, "Green"=74, "Blue"=74}, {"Red"=75, "Green"=75, "Blue"=75}, {"Red"=76, "Green"=76, "Blue"=76}, {"Red"=77, "Green"=77, "Blue"=77}, {"Red"=78, "Green"=78, "Blue"=78}, {"Red"=79, "Green"=79, "Blue"=79}, {"Red"=80, "Green"=80, "Blue"=80}, {"Red"=81, "Green"=81, "Blue"=81}, {"Red"=82, "Green"=82, "Blue"=82}, {"Red"=83, "Green"=83, "Blue"=83}, {"Red"=84, "Green"=84, "Blue"=84}, {"Red"=85, "Green"=85, "Blue"=85}, {"Red"=86, "Green"=86, "Blue"=86}, {"Red"=87, "Green"=87, "Blue"=87}, {"Red"=88, "Green"=88, "Blue"=88}, {"Red"=89, "Green"=89, "Blue"=89}, {"Red"=90, "Green"=90, "Blue"=90}, {"Red"=91, "Green"=91, "Blue"=91}, {"Red"=92, "Green"=92, "Blue"=92}, {"Red"=93, "Green"=93, "Blue"=93}, {"Red"=94, "Green"=94, "Blue"=94}, {"Red"=95, "Green"=95, "Blue"=95}, {"Red"=96, "Green"=96, "Blue"=96}, {"Red"=97, "Green"=97, "Blue"=97}, {"Red"=98, "Green"=98, "Blue"=98}, {"Red"=99, "Green"=99, "Blue"=99}, {"Red"=100, "Green"=100, "Blue"=100}, {"Red"=101, "Green"=101, "Blue"=101}, {"Red"=102, "Green"=102, "Blue"=102}, {"Red"=103, "Green"=103, "Blue"=103}, {"Red"=104, "Green"=104, "Blue"=104}, {"Red"=105, "Green"=105, "Blue"=105}, {"Red"=106, "Green"=106, "Blue"=106}, {"Red"=107, "Green"=107, "Blue"=107}, {"Red"=108, "Green"=108, "Blue"=108}, {"Red"=109, "Green"=109, "Blue"=109}, {"Red"=110, "Green"=110, "Blue"=110}, {"Red"=111, "Green"=111, "Blue"=111}, {"Red"=112, "Green"=112, "Blue"=112}, {"Red"=113, "Green"=113, "Blue"=113}, {"Red"=114, "Green"=114, "Blue"=114}, {"Red"=115, "Green"=115, "Blue"=115}, {"Red"=116, "Green"=116, "Blue"=116}, {"Red"=117, "Green"=117, "Blue"=117}, {"Red"=118, "Green"=118, "Blue"=118}, {"Red"=119, "Green"=119, "Blue"=119}, {"Red"=120, "Green"=120, "Blue"=120}, {"Red"=121, "Green"=121, "Blue"=121}, {"Red"=122, "Green"=122, "Blue"=122}, {"Red"=123, "Green"=123, "Blue"=123}, {"Red"=124, "Green"=124, "Blue"=124}, {"Red"=125, "Green"=125, "Blue"=125}, {"Red"=126, "Green"=126, "Blue"=126}, {"Red"=127, "Green"=127, "Blue"=127}, {"Red"=128, "Green"=128, "Blue"=128}, {"Red"=129, "Green"=129, "Blue"=129}, {"Red"=130, "Green"=130, "Blue"=130}, {"Red"=131, "Green"=131, "Blue"=131}, {"Red"=132, "Green"=132, "Blue"=132}, {"Red"=133, "Green"=133, "Blue"=133}, {"Red"=134, "Green"=134, "Blue"=134}, {"Red"=135, "Green"=135, "Blue"=135}, {"Red"=136, "Green"=136, "Blue"=136}, {"Red"=137, "Green"=137, "Blue"=137}, {"Red"=138, "Green"=138, "Blue"=138}, {"Red"=139, "Green"=139, "Blue"=139}, {"Red"=140, "Green"=140, "Blue"=140}, {"Red"=141, "Green"=141, "Blue"=141}, {"Red"=142, "Green"=142, "Blue"=142}, {"Red"=143, "Green"=143, "Blue"=143}, {"Red"=144, "Green"=144, "Blue"=144}, {"Red"=145, "Green"=145, "Blue"=145}, {"Red"=146, "Green"=146, "Blue"=146}, {"Red"=147, "Green"=147, "Blue"=147}, {"Red"=148, "Green"=148, "Blue"=148}, {"Red"=149, "Green"=149, "Blue"=149}, {"Red"=150, "Green"=150, "Blue"=150}, {"Red"=151, "Green"=151, "Blue"=151}, {"Red"=152, "Green"=152, "Blue"=152}, {"Red"=153, "Green"=153, "Blue"=153}, {"Red"=154, "Green"=154, "Blue"=154}, {"Red"=155, "Green"=155, "Blue"=155}, {"Red"=156, "Green"=156, "Blue"=156}, {"Red"=157, "Green"=157, "Blue"=157}, {"Red"=158, "Green"=158, "Blue"=158}, {"Red"=159, "Green"=159, "Blue"=159}, {"Red"=160, "Green"=160, "Blue"=160}, {"Red"=161, "Green"=161, "Blue"=161}, {"Red"=162, "Green"=162, "Blue"=162}, {"Red"=163, "Green"=163, "Blue"=163}, {"Red"=164, "Green"=164, "Blue"=164}, {"Red"=165, "Green"=165, "Blue"=165}, {"Red"=166, "Green"=166, "Blue"=166}, {"Red"=167, "Green"=167, "Blue"=167}, {"Red"=168, "Green"=168, "Blue"=168}, {"Red"=169, "Green"=169, "Blue"=169}, {"Red"=170, "Green"=170, "Blue"=170}, {"Red"=171, "Green"=171, "Blue"=171}, {"Red"=172, "Green"=172, "Blue"=172}, {"Red"=173, "Green"=173, "Blue"=173}, {"Red"=174, "Green"=174, "Blue"=174}, {"Red"=175, "Green"=175, "Blue"=175}, {"Red"=176, "Green"=176, "Blue"=176}, {"Red"=177, "Green"=177, "Blue"=177}, {"Red"=178, "Green"=178, "Blue"=178}, {"Red"=179, "Green"=179, "Blue"=179}, {"Red"=180, "Green"=180, "Blue"=180}, {"Red"=181, "Green"=181, "Blue"=181}, {"Red"=182, "Green"=182, "Blue"=182}, {"Red"=183, "Green"=183, "Blue"=183}, {"Red"=184, "Green"=184, "Blue"=184}, {"Red"=185, "Green"=185, "Blue"=185}, {"Red"=186, "Green"=186, "Blue"=186}, {"Red"=187, "Green"=187, "Blue"=187}, {"Red"=188, "Green"=188, "Blue"=188}, {"Red"=189, "Green"=189, "Blue"=189}, {"Red"=190, "Green"=190, "Blue"=190}, {"Red"=191, "Green"=191, "Blue"=191}, {"Red"=192, "Green"=192, "Blue"=192}, {"Red"=193, "Green"=193, "Blue"=193}, {"Red"=194, "Green"=194, "Blue"=194}, {"Red"=195, "Green"=195, "Blue"=195}, {"Red"=196, "Green"=196, "Blue"=196}, {"Red"=197, "Green"=197, "Blue"=197}, {"Red"=198, "Green"=198, "Blue"=198}, {"Red"=199, "Green"=199, "Blue"=199}, {"Red"=200, "Green"=200, "Blue"=200}, {"Red"=201, "Green"=201, "Blue"=201}, {"Red"=202, "Green"=202, "Blue"=202}, {"Red"=203, "Green"=203, "Blue"=203}, {"Red"=204, "Green"=204, "Blue"=204}, {"Red"=205, "Green"=205, "Blue"=205}, {"Red"=206, "Green"=206, "Blue"=206}, {"Red"=207, "Green"=207, "Blue"=207}, {"Red"=208, "Green"=208, "Blue"=208}, {"Red"=209, "Green"=209, "Blue"=209}, {"Red"=210, "Green"=210, "Blue"=210}, {"Red"=211, "Green"=211, "Blue"=211}, {"Red"=212, "Green"=212, "Blue"=212}, {"Red"=213, "Green"=213, "Blue"=213}, {"Red"=214, "Green"=214, "Blue"=214}, {"Red"=215, "Green"=215, "Blue"=215}, {"Red"=216, "Green"=216, "Blue"=216}, {"Red"=217, "Green"=217, "Blue"=217}, {"Red"=218, "Green"=218, "Blue"=218}, {"Red"=219, "Green"=219, "Blue"=219}, {"Red"=220, "Green"=220, "Blue"=220}, {"Red"=221, "Green"=221, "Blue"=221}, {"Red"=222, "Green"=222, "Blue"=222}, {"Red"=223, "Green"=223, "Blue"=223}, {"Red"=224, "Green"=224, "Blue"=224}, {"Red"=225, "Green"=225, "Blue"=225}, {"Red"=226, "Green"=226, "Blue"=226}, {"Red"=227, "Green"=227, "Blue"=227}, {"Red"=228, "Green"=228, "Blue"=228}, {"Red"=229, "Green"=229, "Blue"=229}, {"Red"=230, "Green"=230, "Blue"=230}, {"Red"=231, "Green"=231, "Blue"=231}, {"Red"=232, "Green"=232, "Blue"=232}, {"Red"=233, "Green"=233, "Blue"=233}, {"Red"=234, "Green"=234, "Blue"=234}, {"Red"=235, "Green"=235, "Blue"=235}, {"Red"=236, "Green"=236, "Blue"=236}, {"Red"=237, "Green"=237, "Blue"=237}, {"Red"=238, "Green"=238, "Blue"=238}, {"Red"=239, "Green"=239, "Blue"=239}, {"Red"=240, "Green"=240, "Blue"=240}, {"Red"=241, "Green"=241, "Blue"=241}, {"Red"=242, "Green"=242, "Blue"=242}, {"Red"=243, "Green"=243, "Blue"=243}, {"Red"=244, "Green"=244, "Blue"=244}, {"Red"=245, "Green"=245, "Blue"=245}, {"Red"=246, "Green"=246, "Blue"=246}, {"Red"=247, "Green"=247, "Blue"=247}, {"Red"=248, "Green"=248, "Blue"=248}, {"Red"=249, "Green"=249, "Blue"=249}, {"Red"=250, "Green"=250, "Blue"=250}, {"Red"=251, "Green"=251, "Blue"=251}, {"Red"=252, "Green"=252, "Blue"=252}, {"Red"=253, "Green"=253, "Blue"=253}, {"Red"=254, "Green"=254, "Blue"=254}, {"Red"=255, "Green"=0, "Blue"=0}] ("Color Palette") cluster{"Red":u8, "Green":u8, "Blue":u8}[] [{"Red"=0, "Green"=0, "Blue"=0}, {"Red"=1, "Green"=1, "Blue"=1}, {"Red"=2, "Green"=2, "Blue"=2}, {"Red"=3, "Green"=3, "Blue"=3}, {"Red"=4, "Green"=4, "Blue"=4}, {"Red"=5, "Green"=5, "Blue"=5}, {"Red"=6, "Green"=6, "Blue"=6}, {"Red"=7, "Green"=7, "Blue"=7}, {"Red"=8, "Green"=8, "Blue"=8}, {"Red"=9, "Green"=9, "Blue"=9}, {"Red"=10, "Green"=10, "Blue"=10}, {"Red"=11, "Green"=11, "Blue"=11}, {"Red"=12, "Green"=12, "Blue"=12}, {"Red"=13, "Green"=13, "Blue"=13}, {"Red"=14, "Green"=14, "Blue"=14}, {"Red"=15, "Green"=15, "Blue"=15}, {"Red"=16, "Green"=16, "Blue"=16}, {"Red"=17, "Green"=17, "Blue"=17}, {"Red"=18, "Green"=18, "Blue"=18}, {"Red"=19, "Green"=19, "Blue"=19}, {"Red"=20, "Green"=20, "Blue"=20}, {"Red"=21, "Green"=21, "Blue"=21}, {"Red"=22, "Green"=22, "Blue"=22}, {"Red"=23, "Green"=23, "Blue"=23}, {"Red"=24, "Green"=24, "Blue"=24}, {"Red"=25, "Green"=25, "Blue"=25}, {"Red"=26, "Green"=26, "Blue"=26}, {"Red"=27, "Green"=27, "Blue"=27}, {"Red"=28, "Green"=28, "Blue"=28}, {"Red"=29, "Green"=29, "Blue"=29}, {"Red"=30, "Green"=30, "Blue"=30}, {"Red"=31, "Green"=31, "Blue"=31}, {"Red"=32, "Green"=32, "Blue"=32}, {"Red"=33, "Green"=33, "Blue"=33}, {"Red"=34, "Green"=34, "Blue"=34}, {"Red"=35, "Green"=35, "Blue"=35}, {"Red"=36, "Green"=36, "Blue"=36}, {"Red"=37, "Green"=37, "Blue"=37}, {"Red"=38, "Green"=38, "Blue"=38}, {"Red"=39, "Green"=39, "Blue"=39}, {"Red"=40, "Green"=40, "Blue"=40}, {"Red"=41, "Green"=41, "Blue"=41}, {"Red"=42, "Green"=42, "Blue"=42}, {"Red"=43, "Green"=43, "Blue"=43}, {"Red"=44, "Green"=44, "Blue"=44}, {"Red"=45, "Green"=45, "Blue"=45}, {"Red"=46, "Green"=46, "Blue"=46}, {"Red"=47, "Green"=47, "Blue"=47}, {"Red"=48, "Green"=48, "Blue"=48}, {"Red"=49, "Green"=49, "Blue"=49}, {"Red"=50, "Green"=50, "Blue"=50}, {"Red"=51, "Green"=51, "Blue"=51}, {"Red"=52, "Green"=52, "Blue"=52}, {"Red"=53, "Green"=53, "Blue"=53}, {"Red"=54, "Green"=54, "Blue"=54}, {"Red"=55, "Green"=55, "Blue"=55}, {"Red"=56, "Green"=56, "Blue"=56}, {"Red"=57, "Green"=57, "Blue"=57}, {"Red"=58, "Green"=58, "Blue"=58}, {"Red"=59, "Green"=59, "Blue"=59}, {"Red"=60, "Green"=60, "Blue"=60}, {"Red"=61, "Green"=61, "Blue"=61}, {"Red"=62, "Green"=62, "Blue"=62}, {"Red"=63, "Green"=63, "Blue"=63}, {"Red"=64, "Green"=64, "Blue"=64}, {"Red"=65, "Green"=65, "Blue"=65}, {"Red"=66, "Green"=66, "Blue"=66}, {"Red"=67, "Green"=67, "Blue"=67}, {"Red"=68, "Green"=68, "Blue"=68}, {"Red"=69, "Green"=69, "Blue"=69}, {"Red"=70, "Green"=70, "Blue"=70}, {"Red"=71, "Green"=71, "Blue"=71}, {"Red"=72, "Green"=72, "Blue"=72}, {"Red"=73, "Green"=73, "Blue"=73}, {"Red"=74, "Green"=74, "Blue"=74}, {"Red"=75, "Green"=75, "Blue"=75}, {"Red"=76, "Green"=76, "Blue"=76}, {"Red"=77, "Green"=77, "Blue"=77}, {"Red"=78, "Green"=78, "Blue"=78}, {"Red"=79, "Green"=79, "Blue"=79}, {"Red"=80, "Green"=80, "Blue"=80}, {"Red"=81, "Green"=81, "Blue"=81}, {"Red"=82, "Green"=82, "Blue"=82}, {"Red"=83, "Green"=83, "Blue"=83}, {"Red"=84, "Green"=84, "Blue"=84}, {"Red"=85, "Green"=85, "Blue"=85}, {"Red"=86, "Green"=86, "Blue"=86}, {"Red"=87, "Green"=87, "Blue"=87}, {"Red"=88, "Green"=88, "Blue"=88}, {"Red"=89, "Green"=89, "Blue"=89}, {"Red"=90, "Green"=90, "Blue"=90}, {"Red"=91, "Green"=91, "Blue"=91}, {"Red"=92, "Green"=92, "Blue"=92}, {"Red"=93, "Green"=93, "Blue"=93}, {"Red"=94, "Green"=94, "Blue"=94}, {"Red"=95, "Green"=95, "Blue"=95}, {"Red"=96, "Green"=96, "Blue"=96}, {"Red"=97, "Green"=97, "Blue"=97}, {"Red"=98, "Green"=98, "Blue"=98}, {"Red"=99, "Green"=99, "Blue"=99}, {"Red"=100, "Green"=100, "Blue"=100}, {"Red"=101, "Green"=101, "Blue"=101}, {"Red"=102, "Green"=102, "Blue"=102}, {"Red"=103, "Green"=103, "Blue"=103}, {"Red"=104, "Green"=104, "Blue"=104}, {"Red"=105, "Green"=105, "Blue"=105}, {"Red"=106, "Green"=106, "Blue"=106}, {"Red"=107, "Green"=107, "Blue"=107}, {"Red"=108, "Green"=108, "Blue"=108}, {"Red"=109, "Green"=109, "Blue"=109}, {"Red"=110, "Green"=110, "Blue"=110}, {"Red"=111, "Green"=111, "Blue"=111}, {"Red"=112, "Green"=112, "Blue"=112}, {"Red"=113, "Green"=113, "Blue"=113}, {"Red"=114, "Green"=114, "Blue"=114}, {"Red"=115, "Green"=115, "Blue"=115}, {"Red"=116, "Green"=116, "Blue"=116}, {"Red"=117, "Green"=117, "Blue"=117}, {"Red"=118, "Green"=118, "Blue"=118}, {"Red"=119, "Green"=119, "Blue"=119}, {"Red"=120, "Green"=120, "Blue"=120}, {"Red"=121, "Green"=121, "Blue"=121}, {"Red"=122, "Green"=122, "Blue"=122}, {"Red"=123, "Green"=123, "Blue"=123}, {"Red"=124, "Green"=124, "Blue"=124}, {"Red"=125, "Green"=125, "Blue"=125}, {"Red"=126, "Green"=126, "Blue"=126}, {"Red"=127, "Green"=127, "Blue"=127}, {"Red"=128, "Green"=128, "Blue"=128}, {"Red"=129, "Green"=129, "Blue"=129}, {"Red"=130, "Green"=130, "Blue"=130}, {"Red"=131, "Green"=131, "Blue"=131}, {"Red"=132, "Green"=132, "Blue"=132}, {"Red"=133, "Green"=133, "Blue"=133}, {"Red"=134, "Green"=134, "Blue"=134}, {"Red"=135, "Green"=135, "Blue"=135}, {"Red"=136, "Green"=136, "Blue"=136}, {"Red"=137, "Green"=137, "Blue"=137}, {"Red"=138, "Green"=138, "Blue"=138}, {"Red"=139, "Green"=139, "Blue"=139}, {"Red"=140, "Green"=140, "Blue"=140}, {"Red"=141, "Green"=141, "Blue"=141}, {"Red"=142, "Green"=142, "Blue"=142}, {"Red"=143, "Green"=143, "Blue"=143}, {"Red"=144, "Green"=144, "Blue"=144}, {"Red"=145, "Green"=145, "Blue"=145}, {"Red"=146, "Green"=146, "Blue"=146}, {"Red"=147, "Green"=147, "Blue"=147}, {"Red"=148, "Green"=148, "Blue"=148}, {"Red"=149, "Green"=149, "Blue"=149}, {"Red"=150, "Green"=150, "Blue"=150}, {"Red"=151, "Green"=151, "Blue"=151}, {"Red"=152, "Green"=152, "Blue"=152}, {"Red"=153, "Green"=153, "Blue"=153}, {"Red"=154, "Green"=154, "Blue"=154}, {"Red"=155, "Green"=155, "Blue"=155}, {"Red"=156, "Green"=156, "Blue"=156}, {"Red"=157, "Green"=157, "Blue"=157}, {"Red"=158, "Green"=158, "Blue"=158}, {"Red"=159, "Green"=159, "Blue"=159}, {"Red"=160, "Green"=160, "Blue"=160}, {"Red"=161, "Green"=161, "Blue"=161}, {"Red"=162, "Green"=162, "Blue"=162}, {"Red"=163, "Green"=163, "Blue"=163}, {"Red"=164, "Green"=164, "Blue"=164}, {"Red"=165, "Green"=165, "Blue"=165}, {"Red"=166, "Green"=166, "Blue"=166}, {"Red"=167, "Green"=167, "Blue"=167}, {"Red"=168, "Green"=168, "Blue"=168}, {"Red"=169, "Green"=169, "Blue"=169}, {"Red"=170, "Green"=170, "Blue"=170}, {"Red"=171, "Green"=171, "Blue"=171}, {"Red"=172, "Green"=172, "Blue"=172}, {"Red"=173, "Green"=173, "Blue"=173}, {"Red"=174, "Green"=174, "Blue"=174}, {"Red"=175, "Green"=175, "Blue"=175}, {"Red"=176, "Green"=176, "Blue"=176}, {"Red"=177, "Green"=177, "Blue"=177}, {"Red"=178, "Green"=178, "Blue"=178}, {"Red"=179, "Green"=179, "Blue"=179}, {"Red"=180, "Green"=180, "Blue"=180}, {"Red"=181, "Green"=181, "Blue"=181}, {"Red"=182, "Green"=182, "Blue"=182}, {"Red"=183, "Green"=183, "Blue"=183}, {"Red"=184, "Green"=184, "Blue"=184}, {"Red"=185, "Green"=185, "Blue"=185}, {"Red"=186, "Green"=186, "Blue"=186}, {"Red"=187, "Green"=187, "Blue"=187}, {"Red"=188, "Green"=188, "Blue"=188}, {"Red"=189, "Green"=189, "Blue"=189}, {"Red"=190, "Green"=190, "Blue"=190}, {"Red"=191, "Green"=191, "Blue"=191}, {"Red"=192, "Green"=192, "Blue"=192}, {"Red"=193, "Green"=193, "Blue"=193}, {"Red"=194, "Green"=194, "Blue"=194}, {"Red"=195, "Green"=195, "Blue"=195}, {"Red"=196, "Green"=196, "Blue"=196}, {"Red"=197, "Green"=197, "Blue"=197}, {"Red"=198, "Green"=198, "Blue"=198}, {"Red"=199, "Green"=199, "Blue"=199}, {"Red"=200, "Green"=200, "Blue"=200}, {"Red"=201, "Green"=201, "Blue"=201}, {"Red"=202, "Green"=202, "Blue"=202}, {"Red"=203, "Green"=203, "Blue"=203}, {"Red"=204, "Green"=204, "Blue"=204}, {"Red"=205, "Green"=205, "Blue"=205}, {"Red"=206, "Green"=206, "Blue"=206}, {"Red"=207, "Green"=207, "Blue"=207}, {"Red"=208, "Green"=208, "Blue"=208}, {"Red"=209, "Green"=209, "Blue"=209}, {"Red"=210, "Green"=210, "Blue"=210}, {"Red"=211, "Green"=211, "Blue"=211}, {"Red"=212, "Green"=212, "Blue"=212}, {"Red"=213, "Green"=213, "Blue"=213}, {"Red"=214, "Green"=214, "Blue"=214}, {"Red"=215, "Green"=215, "Blue"=215}, {"Red"=216, "Green"=216, "Blue"=216}, {"Red"=217, "Green"=217, "Blue"=217}, {"Red"=218, "Green"=218, "Blue"=218}, {"Red"=219, "Green"=219, "Blue"=219}, {"Red"=220, "Green"=220, "Blue"=220}, {"Red"=221, "Green"=221, "Blue"=221}, {"Red"=222, "Green"=222, "Blue"=222}, {"Red"=223, "Green"=223, "Blue"=223}, {"Red"=224, "Green"=224, "Blue"=224}, {"Red"=225, "Green"=225, "Blue"=225}, {"Red"=226, "Green"=226, "Blue"=226}, {"Red"=227, "Green"=227, "Blue"=227}, {"Red"=228, "Green"=228, "Blue"=228}, {"Red"=229, "Green"=229, "Blue"=229}, {"Red"=230, "Green"=230, "Blue"=230}, {"Red"=231, "Green"=231, "Blue"=231}, {"Red"=232, "Green"=232, "Blue"=232}, {"Red"=233, "Green"=233, "Blue"=233}, {"Red"=234, "Green"=234, "Blue"=234}, {"Red"=235, "Green"=235, "Blue"=235}, {"Red"=236, "Green"=236, "Blue"=236}, {"Red"=237, "Green"=237, "Blue"=237}, {"Red"=238, "Green"=238, "Blue"=238}, {"Red"=239, "Green"=239, "Blue"=239}, {"Red"=240, "Green"=240, "Blue"=240}, {"Red"=241, "Green"=241, "Blue"=241}, {"Red"=242, "Green"=242, "Blue"=242}, {"Red"=243, "Green"=243, "Blue"=243}, {"Red"=244, "Green"=244, "Blue"=244}, {"Red"=245, "Green"=245, "Blue"=245}, {"Red"=246, "Green"=246, "Blue"=246}, {"Red"=247, "Green"=247, "Blue"=247}, {"Red"=248, "Green"=248, "Blue"=248}, {"Red"=249, "Green"=249, "Blue"=249}, {"Red"=250, "Green"=250, "Blue"=250}, {"Red"=251, "Green"=251, "Blue"=251}, {"Red"=252, "Green"=252, "Blue"=252}, {"Red"=253, "Green"=253, "Blue"=253}, {"Red"=254, "Green"=254, "Blue"=254}, {"Red"=255, "Green"=255, "Blue"=255}] ("Color Palette")] -> w11
        frame "high clipping red" {
        }
        frame "low clipping blue" {
        }
        frame "high and low clipping" {
        }
        frame "standard", "high / low (full range)" {
        }
      }
      n6 = for {
        tunnel: w16 -> [w30] mode=indexing
        tunnel: w11 -> [w24]
        tunnel: w15 -> [w25]
        tunnel: w19 -> [w26]
        tunnel: [w27] -> _
        tunnel: w17 -> [w29]
        n7 = To More Specific Class(target class=w29, reference=w30) -> (specific class reference=w28:refnum<vi>)  [unwired: 1 in, 1 out]
        n8 = property class="ImageControl"(reference=w28, error in=w26, "User Palette"=w24, "Palette Type"=w25) -> (error out=w27:errorcluster)  [unwired: 1 out]
      }
    }
    frame "display.queue.to.fp.display_MD.completed", "galvo.scan.engine_MD.completed", "image.queue.to.disk.and.display.queue_MD.completed", "raw.queue.to.image.queue_MD.completed" {
      w34 = 2500.0 ("y")
      w52 = 2.0  # two frames at once
      n9 = feedback #1() -> (w37:u32)  [unwired: 1 in]
      "Maximum time delay observed" <- w37
      n10 = call-poly "GFGpolyGet.vi"("Variable Name in"="y.pixels") -> ("Numeric"=w45:dbl)  [unwired: 8 in, 2 out]
      n11 = for {
        N: 1 -> [_]
        shift-right: [w85] -> _
        shift-left: _ -> [w87]
        tunnel: [w86] -> w39
        n12 = Tick Count (ms)() -> (millisecond timer value=w85:u32)
        n13 = Subtract(x=w85, y=w87) -> (x-y=w86:u32)
      }
      n14 = call-poly "GFGpolyGet.vi"("Variable Name in"="x.pixels") -> ("Numeric"=w46:dbl)  [unwired: 8 in, 2 out]
      n15 = call-poly "GFGpolyGet.vi"("Variable Name in"="pixel.dwell.time.in.sec" ("Tag in")) -> ("Numeric"=w44:dbl)  [unwired: 8 in, 2 out]
      n16 = Compound Arithmetic op=MULTIPLY(w46, w45, w44) -> (w43:dbl)
      n17 = First Call?() -> (First Call?: T/F=w41:bool)
      n18 = case shown="False" w41 {
        tunnel: [w81 u32 0] -> w40
        tunnel: w39 -> [w81 _]
        frame False {
        }
        frame True {
        }
      }
      n19 = Multiply(x=w43, y=w52) -> (x*y=w51:dbl)
      n20 = Multiply(x=w51, y=2500.0) -> (x*y=w35:dbl)
      n21 = Greater?(x=w35, y=w34) -> (0:w36:bool)
      n22 = Select(t=w35, s=w36, f=w34) -> (s? t:f=w33:dbl)
      n23 = Greater?(x=w40, y=w37) -> (0:w42:bool)
      n24 = case shown="False" w42 {
        tunnel: w40 -> [_ w84]
        tunnel: [w83 w84] -> w38
        tunnel: w37 -> [w83 _]
        frame False {
        }
        frame True {
        }
      }
      n25 = feedback-in #1(w38) -> ()
      n26 = Greater?(x=w33, y=w39) -> (0:w57:bool)
      n27 = local read "String"() -> (w56:string)
      n28 = Select(t=w56, s=w57, f="") -> (s? t:f=w58:string)
      n29 = Concatenate Strings(w58, "\r\n", w54) -> (w63:string)
      n30 = local write "String"(w63) -> ()
      n31 = for {
        tunnel: w63 -> [w94]
        tunnel: string[] ["galvo.scan.engine_MD.completed", "raw.queue.to.image.queue_MD.completed", "image.queue.to.disk.and.display.queue_MD.completed", "display.queue.to.fp.display_MD.completed"] ("appended array") -> [w93] mode=indexing
        shift-right: [w89] -> w60
        shift-left: i16 0 -> [w88]
        n32 = Match Pattern(string=w94, regular expression=w93) -> (offset past match=w92:i32)  [unwired: 1 in, 3 out]
        n33 = Greater Or Equal To 0?(x=w92) -> (x >= 0?=w91:bool)
        n34 = Boolean To (0,1)(Boolean=w91) -> (0, 1=w90:i16)
        n35 = Add(x=w90, y=w88) -> (x+y=w89:i16)
      }
      n36 = Equal?(x=w60, y=4) -> (x = y?=w31:bool)
      n37 = case shown="True" w31 {
        selector: w31 -> [_ w66]
        tunnel: [150 0] -> w53
        frame False {
        }
        frame True {
          n38 = local write "String"("") -> ()
          n39 = call "GFG_core.vi"("Variable Name in"="ready for flystart?", "Variant in"=w66, "Action"=enum16{"Init", "Set", "Get"}."Set") -> ()  [unwired: 10 in, 7 out]
          n40 = call "GFG_core.vi"("Variable Name in"="flystop", "Variant in"=FALSE ("x = y?"), "Source VI"="completioncheck", "Action"=enum16{"Init", "Set", "Get"}."Set") -> ()  [unwired: 9 in, 7 out]
          n41 = call "MacroRules_FGV.vi"("MacroRules_FGV_Commands"=MacroRules_FGV_Commands."Get Param and Flags", "Command Name IN"="Record") -> ("Flags"=w69:string[])  [unwired: 5 in, 4 out]
          n42 = for {
            tunnel: w69 -> [w79] mode=indexing
            n43 = call "GFG_core.vi"("Variable Name in"=w79, "Variant in"=TRUE, "Action"=enum16{"Init", "Set", "Get"}."Set") -> ()  [unwired: 10 in, 7 out]
          }
        }
      }
    }
    frame "FOCUS", "Record" {
      n44 = Variant To Data(type=TRUE, Variant=w98) -> (data=w96:bool)  [unwired: 1 in, 1 out]
      n45 = case shown="True" w96 {
        frame False {
        }
        frame True {
          n46 = local write "String"("") -> ()
        }
      }
    }
    frame "ROTATE", "Start.Delay", "external.start.trigger.enable", "fill.fraction", "max.field.of.view", "nomin.x.pixels", "pixel.dwell.time.in.sec", "rotate.enable", "voltage.for.max.field.of.view", "x.bidirectional", "x.volt.offset", "y.bidirectional", "y.pixels", "y.volt.offset" {
      n47 = case shown="True" w100 {
        tunnel: w106 -> [_ w112]
        tunnel: w105 -> [_ w111]
        tunnel: w104 -> [_ w110]
        tunnel: w102 -> [_ w109]
        tunnel: w101 -> [_ w107]
        frame False {
        }
        frame True {
          n48 = case shown="\"max.field.of.view\", \"voltage.for.max.field.of.view\"" w107 {
            frame "False", Default {
            }
            frame "max.field.of.view", "voltage.for.max.field.of.view" {
              n49 = call-poly "GFGpolyGet.vi"("Variable Name in"="active.objective") -> ("Numeric"=w175:dbl)  [unwired: 8 in, 2 out]
              n50 = Build Array("max.field.of.view", "voltage.for.max.field.of.view") -> (w180:string[])
              n51 = To Byte Integer(number=w175) -> (8bit integer=w173:i8)
              n52 = Increment(x=w173) -> (x+1=w176:i8)
              n53 = Number To Decimal String(number=w176) -> (decimal integer string=w174:string)  [unwired: 1 in]
              n54 = for {
                tunnel: w180 -> [w188] mode=indexing
                tunnel: w174 -> [w191]
                tunnel: "obj" -> [w192]
                tunnel: "." -> [w190]
                n55 = Concatenate Strings(w192, w191, w190, w188) -> (w189:string)
                n56 = Build Array(w189, w188) -> (w184:string[])
                n57 = Build Array(enum16{"Init", "Set", "Get"}."Get" ("Action"), enum16{"Init", "Set", "Get"}."Set" ("Action")) -> (w185:enum16{"Init", "Set", "Get"}[])
                n58 = Reverse 1D Array(array=w184) -> (reversed array=w183:string[])
                n59 = for {
                  tunnel: w185 -> [w196] mode=indexing
                  tunnel: w183 -> [w195] mode=indexing
                  shift-right: [w194] -> _
                  shift-left: _ -> [w193]
                  n60 = call "GFG_core.vi"("Variable Name in"=w195, "Variant in"=w193, "Action"=w196) -> ("Variant Out"=w194:variant)  [unwired: 10 in, 6 out]
                }
              }
            }
          }
          n61 = case shown="True" w109 {
            tunnel: [_ w114] -> w108
            tunnel: w107 -> [_ w115]
            frame False {
            }
            frame True {
              n62 = call-poly "GFGpolyGet.vi"("Variable Name in"=w115) -> ("output cluster"=w117:T15)  [unwired: 9 in, 1 out]
              n63 = Unbundle(w117) -> ("WaveformChartRef"=w121:refnum<vi>, "DigitalRef"=w122:refnum<vi>, "ArrayRef"=w123:refnum<vi>, "TabControlRef"=w124:refnum<vi>, "EnumRef"=w125:refnum<vi>, "RingRef"=w126:refnum<vi>, "BooleanRef"=w127:refnum<vi>, "KnobRef"=w128:refnum<vi>, "SlideRef"=w129:refnum<vi>, "PathRef"=w130:refnum<vi>, "StringRef"=w131:refnum<vi>, "ComboBox"=w120:refnum<vi>, "WaveformGraphRef"=w119:refnum<vi>)
              n64 = Build Array(w121, w122, w123, w124, w125, w126, w127, w128, w129, w130, w131, w120, w119) -> (w118:refnum<vi>[])
              n65 = for {
                tunnel: w118 -> [w143] mode=indexing
                tunnel: [w143] -> w116
                stop <- w144 continue-if-true
                n66 = Not A Number/Path/Refnum?(number/path/refnum=w143) -> (NaN/Path/Refnum?=w144:bool)
              }
              n67 = call "wait for fp element value stable.vi"("CtlRef"=w116) -> ("error out"=w113:errorcluster)  [unwired: 9 in, 1 out]
              n68 = flat-sequence {
                tunnel: [w134] -> w132
                tunnel: [w135] -> w114
                tunnel: w113 -> [_]
                frame #0 {
                  n69 = call-poly "GFGpolyGet.vi"("Variable Name in"="FOCUS") -> ("Boolean Value OUT"=w141:bool)  [unwired: 9 in, 1 out]
                  n70 = call "Timer.vi"("Timer Command"=Timer_Commands."Check Time", "name qualifier (empty if unwired)"="flystop censor period") -> ("Complete?"=w136:bool)  [unwired: 4 in, 5 out]
                  n71 = And(x=w141, y=w136) -> (x .and. y?=w134:bool)
                  n72 = call "GFG_core.vi"("Variable Name in"="flystop", "Variant in"=w134, "Source VI"="rotatecase", "Action"=enum16{"Init", "Set", "Get"}."Set") -> ("error out"=w135:errorcluster)  [unwired: 9 in, 6 out]
                }
              }
              n73 = case shown="True" w132 {
                tunnel: w114 -> [_ _]
                frame False {
                }
                frame True {
                  n74 = call "kill task and queues for flystart.vi"() -> ()  [unwired: 12 in]
                  n75 = Build Array("Start.Delay" ("Variable Name in"), "ZOOM" ("Variable Name in"), "pixel.resolution" ("element"), "speed.mode" ("element")) -> (w148:string[])
                  n76 = for {
                    tunnel: w148 -> [w170] mode=indexing
                    n77 = call-poly "GFGpolyGet.vi"("Variable Name in"=w170) -> ("output cluster"=w155:T15)  [unwired: 9 in, 1 out]
                    n78 = Unbundle(w155) -> ("WaveformChartRef"=w159:refnum<vi>, "DigitalRef"=w160:refnum<vi>, "ArrayRef"=w161:refnum<vi>, "TabControlRef"=w162:refnum<vi>, "EnumRef"=w163:refnum<vi>, "RingRef"=w164:refnum<vi>, "BooleanRef"=w165:refnum<vi>, "KnobRef"=w166:refnum<vi>, "SlideRef"=w167:refnum<vi>, "PathRef"=w168:refnum<vi>, "StringRef"=w169:refnum<vi>, "ComboBox"=w158:refnum<vi>, "WaveformGraphRef"=w157:refnum<vi>)
                    n79 = Build Array(w159, w160, w161, w162, w163, w164, w165, w166, w167, w168, w169, w158, w157) -> (w156:refnum<vi>[])
                    n80 = for {
                      tunnel: w156 -> [w171] mode=indexing
                      tunnel: [w171] -> w153
                      stop <- w172 continue-if-true
                      n81 = Not A Number/Path/Refnum?(number/path/refnum=w171) -> (NaN/Path/Refnum?=w172:bool)
                    }
                    n82 = property class="Ctl"(reference=w153, "DisabledEnum"=T4."Disabled and Grayed Out" ("Disabled")) -> ()  [unwired: 1 in, 2 out]
                  }
                  n83 = call "Timer.vi"("Timer Command"=Timer_Commands."Start", "name qualifier (empty if unwired)"="flystop censor period", "Set Time IN (s)"=2.0) -> ()  [unwired: 3 in, 6 out]
                }
              }
            }
          }
          n84 = case shown="\"pixel.dwell.time.in.sec.\"" w107 {
            tunnel: w112 -> [_ w238 _ _]
            tunnel: w111 -> [_ _ w261 _]
            tunnel: w110 -> [_ _ _ w268]
            tunnel: w108 -> [_ _ _ _]
            frame "False", Default {
              n85 = call-poly "GFGpolyGet.vi"("Variable Name in"="y.pixels") -> ("Numeric"=w201:dbl)  [unwired: 8 in, 2 out]
              n86 = call-poly "GFGpolyGet.vi"("Variable Name in"="fill.fraction") -> ("Numeric"=w213:dbl)  [unwired: 8 in, 2 out]
              n87 = call-poly "GFGpolyGet.vi"("Variable Name in"="nomin.x.pixels") -> ("Numeric"=w203:dbl)  [unwired: 8 in, 2 out]
              n88 = call "GFG_core.vi"("Variable Name in"="pixel.resolution") -> ("Variant Out"=w198:variant)  [unwired: 12 in, 6 out]
              n89 = Variant To Data(type=pixel_resolution_enum."128 x 128" ("pixel resolution"), Variant=w198) -> (data=w197:T5)  [unwired: 1 in, 1 out]
              n90 = call-poly "GFGpolyGet.vi"("Variable Name in"="max.field.of.view") -> ("Numeric"=w216:dbl)  [unwired: 8 in, 2 out]
              n91 = call-poly "GFGpolyGet.vi"("Variable Name in"="ZOOM") -> ("Numeric"=w215:dbl)  [unwired: 8 in, 2 out]
              n92 = Build Array(w203, w201) -> (w206:dbl[])
              n93 = Divide(x=w213, y=100.0) -> (x/y=w211:dbl)
              n94 = Divide(x=w203, y=w211) -> (x/y=w208:dbl)
              n95 = Divide(x=w216, y=w215) -> (x/y=w207:dbl)
              n96 = Array Max & Min(array=w206) -> (max value=w205:dbl)  [unwired: 3 out]
              n97 = case shown="\"256 x 128\", Default" w197 {
                tunnel: w207 -> [_ w221]
                tunnel: w205 -> [_ w219]
                frame "arbitrary" {
                }
                frame "256 x 128", Default {
                  n98 = Divide(x=w221, y=w219) -> (x/y=w220:dbl)
                  n99 = call "GFG_core.vi"("Variable Name in"="y.pixel.sz", "Variant in"=w220, "Action"=enum16{"Init", "Set", "Get"}."Set") -> ()  [unwired: 10 in, 7 out]
                  n100 = call "GFG_core.vi"("Variable Name in"="x.pixel.sz", "Variant in"=w220, "Action"=enum16{"Init", "Set", "Get"}."Set") -> ()  [unwired: 10 in, 7 out]
                }
              }
              n101 = call "GFG_core.vi"("Variable Name in"="x.pixels", "Variant in"=w208, "Action"=enum16{"Init", "Set", "Get"}."Set") -> ()  [unwired: 10 in, 7 out]
            }
            frame "x.bidirectional" {
              n102 = Variant To Data(type=TRUE, Variant=w238) -> (data=w226:bool)  [unwired: 1 in, 1 out]
              n103 = call-poly "GFGpolyGet.vi"("Variable Name in"="speed mode") -> ("output cluster"=w235:T15)  [unwired: 9 in, 1 out]
              n104 = Unbundle By Name(w235) -> ("RingRef"=w231:refnum<vi>)
              n105 = Select(t=i32[] [] ("Disabled Items []"), s=w226, f=i32[] [0, 1] ("Disabled Items []")) -> (s? t:f=w232:i32[])
              n106 = property class="Ring"(reference=w231) -> (reference out=w227:refnum<vi>, "Value"=w230:variant)  [unwired: 1 in, 1 out]
              n107 = call "GFG_core.vi"("Variable Name in"="scan mode main settings") -> ("Variant Out"=w241:variant)  [unwired: 12 in, 6 out]
              n108 = Variant To Data(type=scan_mode_main_settings_tab."2D line scan" ("scan mode main settings"), Variant=w241) -> (data=w239:T6)  [unwired: 1 in, 1 out]
              n109 = Select(t=w230, s=w226, f=2) -> (s? t:f=w228:variant)
              n110 = case shown="\"2D frame\", Default" w239 {
                tunnel: w226 -> [w248 _]
                frame "2D frame", Default {
                  n111 = call "GFG_core.vi"("Variable Name in"="fill.fraction.bidi") -> ("Variant Out"=w250:variant)  [unwired: 12 in, 6 out]
                  n112 = call-poly "GFGpolyGet.vi"("Variable Name in"="MAIN Image panels ") -> ("output cluster"=w244:T15)  [unwired: 9 in, 1 out]
                  n113 = call "GFG_core.vi"("Variable Name in"="fill.fraction.unidi") -> ("Variant Out"=w251:variant)  [unwired: 12 in, 6 out]
                  n114 = call "GFG refresh all variables.vi"("Variables to refresh"=string[] ["pixel resolution"] ("All Variable Names")) -> ()  [unwired: 11 in]
                  n115 = Unbundle By Name(w244) -> ("TabControlRef"=w246:refnum<vi>)
                  n116 = Select(t=w250, s=w248, f=w251) -> (s? t:f=w249:variant)
                  n117 = property class="TabCtl"(reference=w246, "Tabs Visible?"=TRUE) -> ()  [unwired: 1 in, 2 out]
                  n118 = call "GFG_core.vi"("Variable Name in"="fill.fraction", "Variant in"=w249, "Action"=enum16{"Init", "Set", "Get"}."Set") -> ()  [unwired: 10 in, 7 out]
                }
                frame "2D line scan" {
                  n119 = call "GFG_core.vi"("Variable Name in"="fill.fraction.line", "Action"=enum16{"Init", "Set", "Get"}."Get") -> ("Variant Out"=w256:variant)  [unwired: 11 in, 6 out]
                  n120 = call "GFG_core.vi"("Variable Name in"="fill.fraction", "Variant in"=w256, "Action"=enum16{"Init", "Set", "Get"}."Set") -> ()  [unwired: 10 in, 7 out]
                }
              }
              n121 = property class="Ring"(reference=w227, "Disabled Items []"=w232, "Value"=w228) -> ()  [unwired: 1 in, 2 out]
            }
            frame "pixel.dwell.time.in.sec." {
              n122 = call "GFG_core.vi"("Variable Name in"="scan mode main settings") -> ("Variant Out"=w264:variant)  [unwired: 12 in, 6 out]
              n123 = Variant To Data(type=scan_mode_main_settings_tab."2D line scan" ("scan mode main settings"), Variant=w264) -> (data=w262:T6)  [unwired: 1 in, 1 out]
              n124 = case shown="\"2D frame\", Default" w262 {
                tunnel: [5 w267] -> _
                tunnel: w261 -> [_ w267]
                frame "2D frame", Default {
                }
                frame "2D line scan" {
                }
              }
            }
            frame "fill.fraction" {
              n125 = call "getVIname.vi"() -> ("VI name"=w269:string)  [unwired: 19 in]
              n126 = Not Equal?(x=w269, y=w268) -> (x != y?=w270:bool)
              n127 = case shown="True" w270 {
                frame False {
                }
                frame True {
                  n128 = call "GFG_core.vi"("Variable Name in"="x.bidirectional") -> ("Variant Out"=w277:variant)  [unwired: 12 in, 6 out]
                  n129 = Variant To Data(type=TRUE, Variant=w277) -> (data=w276:bool)  [unwired: 1 in, 1 out]
                  n130 = call "GFG_core.vi"("Variable Name in"="scan mode main settings") -> ("Variant Out"=w274:variant)  [unwired: 12 in, 6 out]
                  n131 = Variant To Data(type=scan_mode_main_settings_tab."2D line scan" ("scan mode main settings"), Variant=w274) -> (data=w271:T6)  [unwired: 1 in, 1 out]
                  n132 = case shown="\"2D frame\", Default" w271 {
                    tunnel: w276 -> [w279 _]
                    frame "2D frame", Default {
                      n133 = case shown="False" w279 {
                        frame False {
                          n134 = call "GFG_core.vi"("Variable Name in"="fill.fraction") -> ("Variant Out"=w280:variant)  [unwired: 12 in, 6 out]
                          n135 = call "GFG_core.vi"("Variable Name in"="fill.fraction.unidi", "Variant in"=w280, "Action"=enum16{"Init", "Set", "Get"}."Set") -> ()  [unwired: 10 in, 7 out]
                        }
                        frame True {
                          n136 = call "GFG_core.vi"("Variable Name in"="fill.fraction") -> ("Variant Out"=w284:variant)  [unwired: 12 in, 6 out]
                          n137 = call "GFG_core.vi"("Variable Name in"="fill.fraction.bidi", "Variant in"=w284, "Action"=enum16{"Init", "Set", "Get"}."Set") -> ()  [unwired: 10 in, 7 out]
                        }
                      }
                    }
                    frame "2D line scan" {
                    }
                  }
                }
              }
            }
          }
        }
      }
    }
    frame "x.pixel.sz", "y.pixel.sz" {
      # "DO NOT DELETE THIS CASE. Needed for resetting timeout value"
    }
    frame "no..of.frames.to.acquire" {
      n138 = feedback #2() -> (w291:variant)  [unwired: 1 in]
      n139 = feedback-in #2(w289) -> ()
      n140 = Not Equal?(x=w289, y=w291) -> (x != y?=w290:bool)
      n141 = case shown="True" w290 {
        frame False {
        }
        frame True {
          n142 = call "calculate tiff files size.vi"() -> ()  [unwired: 11 in, 1 out]
        }
      }
      n143 = call-poly "GFGpolyGet.vi"("Variable Name in"="frame count") -> ("output cluster"=w305:T15)  [unwired: 9 in, 1 out]
      n144 = Unbundle By Name(w305) -> ("SlideRef"=w304:refnum<vi>)
      n145 = Variant To Data(type=0.0, Variant=w289) -> (data=w292:dbl)  [unwired: 1 in, 1 out]
      n146 = call-poly "GFGpolyGet.vi"("Variable Name in"="frames.per.z.cycle") -> ("Numeric"=w296:dbl)  [unwired: 8 in, 2 out]
      n147 = property class="Slide"(reference=w304, "Scale.Maximum"=w292) -> ()  [unwired: 1 in, 2 out]
      n148 = Divide(x=w292, y=w296) -> (x/y=w293:dbl)
      n149 = call "GFG_core.vi"("Variable Name in"="scan mode main settings") -> ("Variant Out"=w300:variant)  [unwired: 12 in, 6 out]
      n150 = Variant To Data(type=scan_mode_main_settings_tab."2D line scan" ("scan mode main settings"), Variant=w300) -> (data=w298:T6)  [unwired: 1 in, 1 out]
      n151 = case shown="\"2D frame\", Default" w298 {
        tunnel: w292 -> [w307 _]
        frame "2D frame", Default {
          n152 = call "GFG_core.vi"("Variable Name in"="no.of.frames.for.frame.scan", "Variant in"=w307, "Action"=enum16{"Init", "Set", "Get"}."Set") -> ()  [unwired: 10 in, 7 out]
        }
        frame "2D line scan" {
        }
      }
      n153 = call "GFG_core.vi"("Variable Name in"="no.of.cycles.to.scan", "Variant in"=w293, "Action"=enum16{"Init", "Set", "Get", "Clear"}."Set") -> ()  [unwired: 10 in, 7 out]
    }
    frame "ai.active0", "ai.active1", "ai.active2", "ai.active3", "file.format" {
      n154 = case shown="\"ai.active0\", \"ai.active1\", \"ai.active2\", \"ai.active3\"" w311 {
        selector: w311 -> [w316 w322]
        tunnel: [w316 w321] -> w310
        frame Default {
        }
        frame "ai.active0", "ai.active1", "ai.active2", "ai.active3" {
          n155 = call-poly "GFGpolyGet.vi"("Variable Name in"="ai.active0") -> ("Boolean Value OUT"=w320:bool)  [unwired: 9 in, 1 out]
          n156 = call-poly "GFGpolyGet.vi"("Variable Name in"="ai.active1") -> ("Boolean Value OUT"=w319:bool)  [unwired: 9 in, 1 out]
          n157 = call-poly "GFGpolyGet.vi"("Variable Name in"="ai.active2") -> ("Boolean Value OUT"=w318:bool)  [unwired: 9 in, 1 out]
          n158 = call-poly "GFGpolyGet.vi"("Variable Name in"="ai.active3") -> ("Boolean Value OUT"=w317:bool)  [unwired: 9 in, 1 out]
          n159 = Boolean To (0,1)(Boolean=w320) -> (0, 1=w323:i16)
          n160 = Boolean To (0,1)(Boolean=w319) -> (0, 1=w324:i16)
          n161 = Boolean To (0,1)(Boolean=w318) -> (0, 1=w325:i16)
          n162 = Boolean To (0,1)(Boolean=w317) -> (0, 1=w326:i16)
          n163 = Compound Arithmetic op=ADD(w323, w324, w325, w326) -> (w327:i16)
          n164 = Equal To 0?(x=w327) -> (x = 0?=w328:bool)
          n165 = case shown="True" w328 {
            tunnel: w322 -> [w333 w335]
            tunnel: [w333 w335] -> w321
            frame False {
            }
            frame True {
              # "undo the change."
              n166 = call "GFG_core.vi"("Variable Name in"=w335, "Variant in"=TRUE ("Value"), "Action"=enum16{"Init", "Set", "Get", "Clear"}."Set") -> ()  [unwired: 10 in, 7 out]
              n167 = One Button Dialog(message="At least one channel must be selected! Please select another channel first to proceed!") -> ()  [unwired: 1 in, 1 out]
            }
          }
        }
      }
      n168 = flat-sequence {
        tunnel: w310 -> [_]
        frame #0 {
          n169 = call "calculate tiff files size.vi"() -> ("no. of channels"=w313:i16)  [unwired: 11 in]
          n170 = call "GFG_core.vi"("Variable Name in"="no.of.channels" ("Tag in"), "Variant in"=w313, "Action"=enum16{"Init", "Set", "Get", "Clear"}."Set") -> ()  [unwired: 10 in, 7 out]
        }
      }
    }
    frame "reset.zoom" {
      n171 = call-poly "GFGpolyGet.vi"() -> ("DisplayRefsOut(generic class)"=w343:T14)  [unwired: 10 in, 1 out]
      n172 = call-poly "GFGpolyGet.vi"() -> ("Image Refs Out"=w342:T17)  [unwired: 10 in, 1 out]
      n173 = Cluster To Array(cluster=w343) -> (array=w341:refnum<vi>[])
      n174 = Cluster To Array(cluster=w342) -> (array=w340:T16[])
      n175 = call "set initial zoom.vi"("reset?"=TRUE, "Image Refs In"=w340, "DisplayRefsIn(generic class)"=w341) -> ()  [unwired: 9 in]
    }
    frame "ZOOM", "pixel.resolution", "speed.mode" {
      # "Check, if speed mode has been changed, whilst FOCUS is active."
      n176 = call-poly "GFGpolyGet.vi"("Variable Name in"="FOCUS") -> ("Boolean Value OUT"=w351:bool)  [unwired: 9 in, 1 out]
      n177 = Equal?(x=w349, y="speed.mode" ("Variable Name in")) -> (x = y?=w348:bool)
      n178 = And(x=w351, y=w348) -> (x .and. y?=w346:bool)
      n179 = case "Check, if there is a speed change on the fly and if it is possible to apply!" shown="True" w346 {
        tunnel: w347 -> [_ w551]
        tunnel: [w549 w552] -> w345
        frame False {
          w549 = TRUE  # Execute regular code, this is not a speed change on the fly!
        }
        frame True {
          w555 = T18 2 items=["extra fast scan", "fast scan", "standard scan", "long exposure"] ("speed mode")
          # "new speed"
          # "current speed"
          # "Check, if the new speed mode would change the pixel dwell time."
          n180 = Variant To Data(type=w555, Variant=w551) -> (data=w556:T18)  [unwired: 1 in, 1 out]
          n181 = call-poly "GFGpolyGet.vi"("Variable Name in"="pixel.dwell.time.in.sec") -> ("Numeric"=w550:dbl)  [unwired: 8 in, 2 out]
          n182 = case shown="0" w556 {
            tunnel: [1e-06 2e-06 4e-06 8e-06] -> w553
            frame 0 {
            }
            frame 1 {
            }
            frame 2, Default {
            }
            frame 3 {
            }
          }
          n183 = Not Equal?(x=w550, y=w553) -> (x != y?=w554:bool)
          n184 = case "Speed change?" shown="True" w554 {
            tunnel: w553 -> [_ w575]
            tunnel: [w562 w564] -> w552
            tunnel: w550 -> [_ w563]
            frame False {
              w562 = FALSE  # No change. Ignore it.
            }
            frame True {
              # "Check for valid scan speed for the x-mirror in a framescan."
              n185 = call-poly "GFGpolyGet.vi"("Variable Name in"="x bidirectional") -> ("Boolean Value OUT"=w577:bool)  [unwired: 9 in, 1 out]
              n186 = call-poly "GFGpolyGet.vi"("Variable Name in"="x.pixels") -> ("Numeric"=w576:dbl)  [unwired: 8 in, 2 out]
              n187 = call-poly "GFGpolyGet.vi"("Variable Name in"="x.speed.limit.in.Hz") -> ("Numeric"=w572:dbl)  [unwired: 8 in, 2 out]
              n188 = Multiply(x=w576, y=w575) -> (x*y=w569:dbl)
              n189 = Reciprocal(x=w569) -> (1/x=w567:dbl)
              n190 = Multiply(x=0.5 ("y"), y=w567) -> (x*y=w570:dbl)
              n191 = Select(t=w570, s=w577, f=w567) -> (s? t:f=w568:dbl)
              n192 = Less?(x=w568, y=w572) -> (x < y?=w565:bool)
              n193 = case shown="False" w565 {
                selector: w565 -> [_ w599]
                tunnel: w568 -> [w598 _]
                tunnel: [w593 w599] -> w564
                tunnel: w563 -> [w581 _]
                frame False {
                  w579 = T18 2 items=["extra fast scan", "fast scan", "standard scan", "long exposure"] ("speed mode")
                  w593 = FALSE  # Invaild! Don't do a flystart!
                  # "Reset speed mode!"
                  n194 = Number To Decimal String(number=w598) -> (decimal integer string=w596:string)  [unwired: 1 in]
                  n195 = Greater?(x=w581, y=1e-06) -> (0:w585:bool)
                  n196 = Greater?(x=w581, y=2e-06) -> (0:w586:bool)
                  n197 = Greater?(x=w581, y=4e-06) -> (0:w587:bool)
                  n198 = Boolean To (0,1)(Boolean=w585) -> (0, 1=w588:i16)
                  n199 = Boolean To (0,1)(Boolean=w586) -> (0, 1=w590:i16)
                  n200 = Boolean To (0,1)(Boolean=w587) -> (0, 1=w589:i16)
                  n201 = Compound Arithmetic op=ADD(w588, w590, w589) -> (w580:i16)
                  n202 = Type Cast(type=w579, x=w580) -> (*(type *) &x=w578:T18)
                  n203 = Concatenate Strings("The current settings would drive the x mirror at " ("message"), w596, "Hz, which is faster than the specified maximum. The scan is running with no changes applied!" ("string")) -> (w594:string)
                  n204 = One Button Dialog(message=w594) -> ()  [unwired: 1 in, 1 out]
                  n205 = call "GFG_core.vi"("Variable Name in"="speed.mode", "Variant in"=w578, "Action"=enum16{"Init", "Set", "Get"}."Set") -> ()  [unwired: 10 in, 7 out]
                }
                frame True {
                  # "Vaild! Apply a flystart as a next step!"
                }
              }
            }
          }
        }
      }
      n206 = case shown="True" w345 {
        tunnel: [w356 120] -> w355
        tunnel: w354 -> [_ w364]
        tunnel: w349 -> [_ w363]
        tunnel: w347 -> [_ w357]
        tunnel: w344 -> [w356 _]
        frame False {
        }
        frame True {
          n207 = case shown="True" w364 {
            tunnel: [_ w368] -> w359
            tunnel: w363 -> [_ w369]
            tunnel: [_ w366] -> w358
            frame False {
            }
            frame True {
              n208 = call-poly "GFGpolyGet.vi"("Variable Name in"=w369) -> ("output cluster"=w371:T15)  [unwired: 9 in, 1 out]
              n209 = Unbundle(w371) -> ("WaveformChartRef"=w375:refnum<vi>, "DigitalRef"=w376:refnum<vi>, "ArrayRef"=w377:refnum<vi>, "TabControlRef"=w378:refnum<vi>, "EnumRef"=w379:refnum<vi>, "RingRef"=w380:refnum<vi>, "BooleanRef"=w381:refnum<vi>, "KnobRef"=w382:refnum<vi>, "SlideRef"=w383:refnum<vi>, "PathRef"=w384:refnum<vi>, "StringRef"=w385:refnum<vi>, "ComboBox"=w374:refnum<vi>, "WaveformGraphRef"=w373:refnum<vi>)
              n210 = Build Array(w375, w376, w377, w378, w379, w380, w381, w382, w383, w384, w385, w374, w373) -> (w372:refnum<vi>[])
              n211 = for {
                tunnel: w372 -> [w396] mode=indexing
                tunnel: [w396] -> w370
                stop <- w397 continue-if-true
                n212 = Not A Number/Path/Refnum?(number/path/refnum=w396) -> (NaN/Path/Refnum?=w397:bool)
              }
              n213 = call "wait for fp element value stable.vi"("CtlRef"=w370) -> ("error out"=w367:errorcluster)  [unwired: 9 in, 1 out]
              n214 = flat-sequence {
                tunnel: [w387] -> w368
                tunnel: w367 -> [_]
                tunnel: [w386] -> w366
                frame #0 {
                  n215 = call-poly "GFGpolyGet.vi"("Variable Name in"="FOCUS") -> ("Boolean Value OUT"=w394:bool)  [unwired: 9 in, 1 out]
                  n216 = call "Timer.vi"("Timer Command"=Timer_Commands."Check Time", "name qualifier (empty if unwired)"="flystop censor period") -> ("Complete?"=w388:bool)  [unwired: 4 in, 5 out]
                  n217 = And(x=w394, y=w388) -> (x .and. y?=w386:bool)
                  n218 = call "GFG_core.vi"("Variable Name in"="flystop", "Variant in"=w386, "Source VI"="zoomcase", "Action"=enum16{"Init", "Set", "Get"}."Set") -> ("error out"=w387:errorcluster)  [unwired: 9 in, 6 out]
                }
              }
              n219 = case shown="True" w366 {
                tunnel: w368 -> [_ _]
                frame False {
                }
                frame True {
                  n220 = Build Array("Start.Delay" ("Variable Name in"), "ZOOM" ("Variable Name in"), "pixel.resolution" ("element"), "speed.mode" ("element")) -> (w401:string[])
                  n221 = call "Timer.vi"("Timer Command"=Timer_Commands."Start", "name qualifier (empty if unwired)"="flystop censor period", "Set Time IN (s)"=2.0) -> ()  [unwired: 3 in, 6 out]
                  n222 = for {
                    tunnel: w401 -> [w423] mode=indexing
                    n223 = call-poly "GFGpolyGet.vi"("Variable Name in"=w423) -> ("output cluster"=w408:T15)  [unwired: 9 in, 1 out]
                    n224 = Unbundle(w408) -> ("WaveformChartRef"=w412:refnum<vi>, "DigitalRef"=w413:refnum<vi>, "ArrayRef"=w414:refnum<vi>, "TabControlRef"=w415:refnum<vi>, "EnumRef"=w416:refnum<vi>, "RingRef"=w417:refnum<vi>, "BooleanRef"=w418:refnum<vi>, "KnobRef"=w419:refnum<vi>, "SlideRef"=w420:refnum<vi>, "PathRef"=w421:refnum<vi>, "StringRef"=w422:refnum<vi>, "ComboBox"=w411:refnum<vi>, "WaveformGraphRef"=w410:refnum<vi>)
                    n225 = Build Array(w412, w413, w414, w415, w416, w417, w418, w419, w420, w421, w422, w411, w410) -> (w409:refnum<vi>[])
                    n226 = for {
                      tunnel: w409 -> [w424] mode=indexing
                      tunnel: [w424] -> w406
                      stop <- w425 continue-if-true
                      n227 = Not A Number/Path/Refnum?(number/path/refnum=w424) -> (NaN/Path/Refnum?=w425:bool)
                    }
                    n228 = property class="Ctl"(reference=w406, "DisabledEnum"=T4."Disabled and Grayed Out" ("Disabled")) -> ()  [unwired: 1 in, 2 out]
                  }
                  n229 = call "kill task and queues for flystart.vi"() -> ()  [unwired: 12 in]
                }
              }
            }
          }
          n230 = case shown="\"pixel.resolution\"" w363 {
            tunnel: w357 -> [_ w431]
            tunnel: [w426 w433] -> w362
            tunnel: w359 -> [_ _]
            tunnel: [_ w430] -> w360
            frame "ZOOM", Default {
              n231 = call "GFG_core.vi"("Variable Name in"="pixel.resolution") -> ("Variant Out"=w428:variant)  [unwired: 12 in, 6 out]
              n232 = Variant To Data(type=pixel_resolution_enum."128 x 128" ("pixel resolution"), Variant=w428) -> (data=w426:T5)  [unwired: 1 in, 1 out]
            }
            frame "pixel.resolution" {
              n233 = feedback #3() -> (w432:variant)  [unwired: 1 in]
              n234 = feedback-in #3(w431) -> ()
              n235 = Not Equal?(x=w431, y=w432) -> (x != y?=w430:bool)
              n236 = Variant To Data(type=pixel_resolution_enum."128 x 128" ("pixel resolution"), Variant=w431) -> (data=w433:T5)  [unwired: 1 in, 1 out]
            }
          }
          n237 = case shown="Default" w362 {
            selector: w362 -> [_ w460]
            tunnel: [_ w458] -> w361
            tunnel: w360 -> [_ w458]
            tunnel: w358 -> [_ w457]
            frame "arbitrary" {
              w439 = "nomin.x.pixels" ("Variable Name in")
              w435 = T4."Disabled and Grayed Out" ("Disabled")
              n238 = call-poly "GFGpolyGet.vi"("Variable Name in"="ZOOM") -> ("output cluster"=w444:T15)  [unwired: 9 in, 1 out]
              n239 = call-poly "GFGpolyGet.vi"("Variable Name in"="speed.mode") -> ("output cluster"=w447:T15)  [unwired: 9 in, 1 out]
              n240 = Unbundle By Name(w444) -> ("SlideRef"=w445:refnum<vi>)
              n241 = call "GFG_core.vi"("Variable Name in"=w439, "Action"=enum16{"Init", "Set", "Get"}."Get") -> ("Variant Out"=w438:variant)  [unwired: 11 in, 6 out]
              n242 = Unbundle By Name(w447) -> ("RingRef"=w446:refnum<vi>)
              n243 = call "GFG_core.vi"("Variable Name in"=w439, "Variant in"=w438, "Action"=enum16{"Init", "Set", "Get"}."Set") -> ()  [unwired: 10 in, 7 out]
              n244 = Build Array("nomin.x.pixels" ("Variable Name in"), "y.pixel.sz" ("Variable Name in"), "x.pixel.sz" ("Variable Name in"), "pixel.dwell.time.in.sec" ("Variable Name in"), "y.pixels" ("Variable Name in")) -> (w448:string[])
              n245 = for {
                tunnel: w448 -> [w455] mode=indexing
                n246 = call-poly "GFGpolyGet.vi"("Variable Name in"=w455) -> ("output cluster"=w454:T15)  [unwired: 9 in, 1 out]
                n247 = Unbundle By Name(w454) -> ("DigitalRef"=w452:refnum<vi>)
                n248 = property class="DigNum"(reference=w452, "DisabledEnum"=T4."Enabled" ("Disabled")) -> ()  [unwired: 1 in, 2 out]
              }
              n249 = property class="Ring"(reference=w446, "DisabledEnum"=w435) -> ()  [unwired: 1 in, 2 out]
              n250 = property class="Slide"(reference=w445, "DisabledEnum"=w435) -> ()  [unwired: 1 in, 2 out]
            }
            frame Default {
              w456 = T18 2 items=["extra fast scan", "fast scan", "standard scan", "long exposure"] ("speed mode")
              n251 = case shown="False" w457 {
                frame False {
                  n252 = Build Array("Start.Delay" ("Variable Name in"), "ZOOM" ("Variable Name in"), "pixel.resolution" ("element"), "speed.mode" ("element")) -> (w497:string[])
                  n253 = for {
                    tunnel: w497 -> [w519] mode=indexing
                    n254 = call-poly "GFGpolyGet.vi"("Variable Name in"=w519) -> ("output cluster"=w504:T15)  [unwired: 9 in, 1 out]
                    n255 = Unbundle(w504) -> ("WaveformChartRef"=w508:refnum<vi>, "DigitalRef"=w509:refnum<vi>, "ArrayRef"=w510:refnum<vi>, "TabControlRef"=w511:refnum<vi>, "EnumRef"=w512:refnum<vi>, "RingRef"=w513:refnum<vi>, "BooleanRef"=w514:refnum<vi>, "KnobRef"=w515:refnum<vi>, "SlideRef"=w516:refnum<vi>, "PathRef"=w517:refnum<vi>, "StringRef"=w518:refnum<vi>, "ComboBox"=w507:refnum<vi>, "WaveformGraphRef"=w506:refnum<vi>)
                    n256 = Build Array(w508, w509, w510, w511, w512, w513, w514, w515, w516, w517, w518, w507, w506) -> (w505:refnum<vi>[])
                    n257 = for {
                      tunnel: w505 -> [w520] mode=indexing
                      tunnel: [w520] -> w502
                      stop <- w521 continue-if-true
                      n258 = Not A Number/Path/Refnum?(number/path/refnum=w520) -> (NaN/Path/Refnum?=w521:bool)
                    }
                    n259 = property class="Ctl"(reference=w502, "DisabledEnum"=T4."Enabled" ("Disabled")) -> ()  [unwired: 1 in, 2 out]
                  }
                }
                frame True {
                }
              }
              n260 = case shown="\"256 x 256\"" w460 {
                tunnel: [128 256 256 512 512 512 512 1024 1024] -> w462
                tunnel: [128 128 256 256 128 64 512 512 1024] -> w461
                frame "128 x 128", Default {
                }
                frame "256 x 128" {
                }
                frame "256 x 256" {
                }
                frame "512 x 256" {
                }
                frame "512 x 128" {
                }
                frame "512 x  64" {
                }
                frame "512 x 512" {
                }
                frame "1024 x 512" {
                }
                frame "1024 x 1024" {
                }
              }
              n261 = call-poly "GFGpolyGet.vi"("Variable Name in"="ZOOM") -> ("Numeric"=w482:dbl)  [unwired: 8 in, 2 out]
              n262 = call-poly "GFGpolyGet.vi"("Variable Name in"="fill.fraction") -> ("Numeric"=w476:dbl)  [unwired: 8 in, 2 out]
              n263 = call-poly "GFGpolyGet.vi"("Variable Name in"="max.field.of.view") -> ("Numeric"=w483:dbl)  [unwired: 8 in, 2 out]
              n264 = Build Array(w462, w461) -> (w468:i32[])
              n265 = Array Max & Min(array=w468) -> (max value=w467:i32)  [unwired: 3 out]
              n266 = call "GFG_core.vi"("Variable Name in"="y.pixels", "Variant in"=w461, "Action"=enum16{"Init", "Set", "Get"}."Set") -> ()  [unwired: 10 in, 7 out]
              n267 = Build Array("nomin.x.pixels" ("Variable Name in"), "y.pixel.sz" ("Variable Name in"), "x.pixel.sz" ("Variable Name in"), "pixel.dwell.time.in.sec" ("Variable Name in"), "y.pixels" ("Variable Name in")) -> (w489:string[])
              n268 = for {
                tunnel: w489 -> [w548] mode=indexing
                n269 = call-poly "GFGpolyGet.vi"("Variable Name in"=w548) -> ("output cluster"=w547:T15)  [unwired: 9 in, 1 out]
                n270 = Unbundle By Name(w547) -> ("DigitalRef"=w545:refnum<vi>)
                n271 = property class="DigNum"(reference=w545, "DisabledEnum"=T4."Disabled and Grayed Out" ("Disabled")) -> (error out=→"error out 2":errorcluster)  [unwired: 1 in, 1 out]
              }
              n272 = Divide(x=w483, y=w482) -> (x/y=w470:dbl)
              n273 = Divide(x=w476, y=100.0) -> (x/y=w474:dbl)
              n274 = Divide(x=w470, y=w467) -> (x/y=w469:dbl)
              n275 = Divide(x=w462, y=w474) -> (x/y=w471:dbl)
              n276 = call "GFG_core.vi"("Variable Name in"="nomin.x.pixels", "Variant in"=w462, "Action"=enum16{"Init", "Set", "Get"}."Set") -> ()  [unwired: 10 in, 7 out]
              n277 = call "GFG_core.vi"("Variable Name in"="x.pixels", "Variant in"=w471, "Action"=enum16{"Init", "Set", "Get"}."Set") -> ()  [unwired: 10 in, 7 out]
              n278 = call "GFG_core.vi"("Variable Name in"="x.pixel.sz", "Variant in"=w469, "Action"=enum16{"Init", "Set", "Get"}."Set") -> ()  [unwired: 10 in, 7 out]
              n279 = call "GFG_core.vi"("Variable Name in"="y.pixel.sz", "Variant in"=w469, "Action"=enum16{"Init", "Set", "Get"}."Set") -> ()  [unwired: 10 in, 7 out]
              n280 = call "GFG_core.vi"("Variable Name in"="speed.mode") -> ("Variant Out"=w487:variant)  [unwired: 12 in, 6 out]
              n281 = Variant To Data(type=w456, Variant=w487) -> (data=w463:T18)  [unwired: 1 in, 1 out]
              n282 = case shown="0" w463 {
                tunnel: [1e-06 2e-06 4e-06 8e-06] -> w464
                frame 0 {
                }
                frame 1 {
                }
                frame 2, Default {
                }
                frame 3 {
                }
              }
              n283 = call "GFG_core.vi"("Variable Name in"="pixel.dwell.time.in.sec", "Variant in"=w464, "Action"=enum16{"Init", "Set", "Get"}."Set") -> ()  [unwired: 10 in, 7 out]
            }
          }
          n284 = case shown="True" w361 {
            frame False {
            }
            frame True {
              n285 = call "calculate tiff files size.vi"() -> ()  [unwired: 11 in, 1 out]
            }
          }
        }
      }
      "Source VI 2" <- w353
    }
    frame "x.invert.image", "y.invert.image" {
    }
    frame "root.path" {
      n286 = disable-structure shown="Disabled" {
        disable-tunnel: w601 -> [w604 _]
        frame Disabled {
          # "Modified by Arjun.\nEarlier, string was being listened to; instead of path"
          n287 = Variant To Data(type=path "" ("path"), Variant=w604) -> (data=w605:path)  [unwired: 1 in, 1 out]
          n288 = Path To String(path=w605) -> (string=w603:string)
          n289 = Search and Replace String(replace all?=TRUE ("replace all? (F)"), input string=w603, search string="[? < > ; ' , * | \" \\t \\r \\n \\s]+", replace string="_" ("replace string (\"\")")) -> (result string=w607:string, number of replacements=w608:i32)  [unwired: 4 in, 2 out]
          "number of replacements" <- w608
          n290 = case shown="1, Default" w608 {
            tunnel: w607 -> [_ w612]
            frame 0 {
            }
            frame 1, Default {
              n291 = String To Path(string=w612) -> (path=w613:path)
              n292 = call "GFG_core.vi"("Variable Name in"="root.path" ("Tag in"), "Variant in"=w613, "Action"=enum16{"Init", "Set", "Get"}."Set") -> ()  [unwired: 10 in, 7 out]
              n293 = Concatenate Strings("Root path contained whitespaces or other disallowed characters.\nThey have been replaced with underscores. The new root path is:\n " ("string"), w612) -> (w616:string)
              n294 = One Button Dialog(message=w616) -> ()  [unwired: 1 in, 1 out]
            }
          }
        }
        frame Enabled {
        }
      }
    }
    frame "custom.step.xy", "custom.step.z" {
      n295 = Variant To Data(type=FALSE, Variant=w619) -> (data=w621:bool)  [unwired: 1 in, 1 out]
      n296 = case shown="True" w621 {
        tunnel: w620 -> [_ w627]
        frame False {
        }
        frame True {
          n297 = case shown="\"custom.step.xy\"" w627 {
            tunnel: [w660 _ w662] -> w626
            tunnel: ["step.size.z" ("Variable Name in") _ "step.size.xy" ("Variable Name in")] -> w632
            frame "custom.step.z" {
              n298 = call "Custom Step Size Z"() -> ("Custom Step Size Z"=w660:dbl)  [unwired: 17 in, 2 out]
            }
            frame Default {
            }
            frame "custom.step.xy" {
              n299 = call "Custom Step Size XY"() -> ("Custom Step Size XY"=w662:dbl)  [unwired: 17 in, 2 out]
            }
          }
          n300 = Equal?(x=w626, y=dbl[] [1.0, 2.0, 5.0, 10.0, 20.0, 50.0]) -> (x = y?=w630:bool[])
          n301 = Less Or Equal To 0?(x=w626) -> (x <= 0?=w623:bool)
          n302 = To Unsigned Word Integer(number=w626) -> (unsigned 16bit integer=w625:u16)
          n303 = Or Array Elements(Boolean array=w630) -> (logical OR=w629:bool)
          n304 = Or(x=w623, y=w629) -> (x .or. y?=w628:bool)
          n305 = case shown="True" w628 {
            tunnel: w632 -> [w647 w648]
            tunnel: w625 -> [w636 w651]
            tunnel: [w636 w653] -> w624
            tunnel: w623 -> [_ w652]
            frame False {
              n306 = call-poly "GFGpolyGet.vi"("Variable Name in"=w647) -> ("output cluster"=w646:T15)  [unwired: 9 in, 1 out]
              n307 = Unbundle By Name(w646) -> ("RingRef"=w645:refnum<vi>)
              n308 = property class="Ring"(reference=w645) -> (reference out=w640:refnum<vi>, "StringsAndValues[]"=w644:T19)  [unwired: 1 in, 1 out]
              n309 = Number To Decimal String(number=w636) -> (decimal integer string=w642:string)  [unwired: 1 in]
              n310 = Array Size(array=w644) -> (size(s)=w637:i32)
              n311 = Decrement(x=w637) -> (x-1=w638:i32)
              n312 = Index Array(array=w644, index=w638) -> (element=w643:cluster{"String":string, "Value":ext})
              n313 = Bundle(cluster=w643, "String"=w642, "Value"=w636) -> (w641:cluster{"String":string, "Value":ext})
              n314 = Replace Array Subset(array=w644, new element=w641, index=w638) -> (w639:T19)
              n315 = property class="Ring"(reference=w640, "StringsAndValues[]"=w639, "Val(Sgnl)"=w636) -> ()  [unwired: 1 in, 2 out]
            }
            frame True {
              # "Ignore values <=0 and standard values, as software would crash with duplicate entries. Entering 100 must be however still possible, as this is the last default value, which always will be repaced by the custom value. To reset it the input 100 must be allowed!"
              n316 = Select(t=u16 0, s=w652, f=w651) -> (s? t:f=w649:u16)
              n317 = case "Switch to existing value" shown="Default" w649 {
                selector: w649 -> [w654 w656]
                tunnel: [w654 w656] -> w653
                tunnel: w648 -> [_ w655]
                frame 0 {
                  # "Ignore values smaller or equal to zero"
                }
                frame Default {
                  n318 = call-poly "GFGpolyGet.vi"("Variable Name in"=w655) -> ("output cluster"=w658:T15)  [unwired: 9 in, 1 out]
                  n319 = Unbundle By Name(w658) -> ("RingRef"=w657:refnum<vi>)
                  n320 = property class="Ring"(reference=w657, "Val(Sgnl)"=w656) -> ()  [unwired: 1 in, 2 out]
                }
              }
            }
          }
          n321 = flat-sequence "Reset pressed button" {
            tunnel: w627 -> [w634]
            tunnel: w624 -> [_]
            frame #0 {
              n322 = call "GFG_core.vi"("Variable Name in"=w634, "Variant in"=FALSE, "Action"=enum16{"Init", "Set", "Get", "Clear"}."Set") -> ()  [unwired: 10 in, 7 out]
            }
          }
        }
      }
    }
    frame "frames.per.z.cycle", "no.of.cycles.to.scan" {
      n323 = call "getVIname.vi"() -> ("VI name"=w664:string)  [unwired: 19 in]
      n324 = Not Equal?(x=w663, y=w664) -> (x != y?=w665:bool)
      n325 = call-poly "GFGpolyGet.vi"("Variable Name in"="x.pixels") -> ("Numeric"=w675:dbl)  [unwired: 8 in, 2 out]
      n326 = call-poly "GFGpolyGet.vi"("Variable Name in"="y.pixels") -> ("Numeric"=w674:dbl)  [unwired: 8 in, 2 out]
      n327 = Multiply(x=w675, y=w674) -> (x*y=w673:dbl)
      n328 = call-poly "GFGpolyGet.vi"("Variable Name in"="pixel.dwell.time.in.sec") -> ("Numeric"=w671:dbl)  [unwired: 8 in, 2 out]
      n329 = call-poly "GFGpolyGet.vi"("Variable Name in"="frames.per.z.cycle") -> ("Numeric"=w666:dbl)  [unwired: 8 in, 2 out]
      n330 = case shown="True" w665 {
        tunnel: w666 -> [_ w681]
        frame False {
        }
        frame True {
          n331 = feedback #4() -> (w686:dbl)  [unwired: 1 in]
          n332 = call-poly "GFGpolyGet.vi"("Variable Name in"="no.of.cycles.to.scan") -> ("Numeric"=w687:dbl)  [unwired: 8 in, 2 out]
          n333 = Greater?(x=w686, y=w687) -> (0:w684:bool)
          n334 = while {
            tunnel: w681 -> [w701]
            shift-right: [w698] -> w683
            shift-left: w687 -> [w695]
            tunnel: 2.0 ("Numeric") -> [w700]
            tunnel: [w697] -> w685
            tunnel: w684 -> [w693]
            stop <- w696 stop-if-true
            n335 = Multiply(x=w701, y=w695) -> (x*y=w697:dbl)
            n336 = Round Toward +Infinity(x=w695) -> (ceil(x): smallest int >= x=w694:dbl)
            n337 = Quotient & Remainder(x=w697, y=w700) -> (x-y*floor(x/y)=w699:dbl)  [unwired: 1 out]
            n338 = Equal To 0?(x=w699) -> (x = 0?=w696:bool)
            n339 = case shown="False" w696 {
              tunnel: w694 -> [w706 w707]
              tunnel: [w702 w707] -> w698
              tunnel: w693 -> [w703 _]
              frame False {
                n340 = Decrement(x=w706) -> (x-1=w705:dbl)
                n341 = Increment(x=w706) -> (x+1=w704:dbl)
                n342 = Select(t=w705, s=w703, f=w704) -> (s? t:f=w702:dbl)
              }
              frame True {
              }
            }
          }
          n343 = feedback-in #4(w683) -> ()
          n344 = call "GFG_core.vi"("Variable Name in"="no. of frames to acquire", "Variant in"=w685, "Action"=enum16{"Init", "Set", "Get", "Clear"}."Set") -> ()  [unwired: 10 in, 7 out]
          n345 = call "GFG_core.vi"("Variable Name in"="no.of.cycles.to.scan", "Variant in"=w683, "Action"=enum16{"Init", "Set", "Get", "Clear"}."Set") -> ()  [unwired: 10 in, 7 out]
        }
      }
      n346 = Multiply(x=w673, y=w671) -> (x*y=w670:dbl)
      n347 = Multiply(x=w666, y=w670) -> (x*y=w669:dbl)
      n348 = Reciprocal(x=w669) -> (1/x=w668:dbl)
      n349 = call "GFG_core.vi"("Variable Name in"="volume rate (in Hz)", "Variant in"=w668, "Action"=enum16{"Init", "Set", "Get", "Clear"}."Set") -> ()  [unwired: 10 in, 7 out]
    }
    frame "scan.mode.main.settings" {
      n350 = Variant To Data(type=scan_mode_main_settings_tab."2D frame" ("scan mode main settings"), Variant=w712) -> (data=w710:T6)  [unwired: 1 in, 1 out]
      n351 = case shown="\"Z Stack\"" w710 {
        tunnel: w709 -> [w749 w780 w787 w808]
        tunnel: [w749 w780 w787 w808] -> w708
        frame "2D frame", Default {
          w714 = enum16{"Init", "Set", "Get"}."Set" ("Action")
          n352 = call-poly "GFGpolyGet.vi"("Variable Name in"="y.pixels") -> ("output cluster"=w740:T15)  [unwired: 9 in, 1 out]
          n353 = Unbundle By Name(w740) -> ("DigitalRef"=w739:refnum<vi>)
          n354 = call-poly "GFGpolyGet.vi"("Variable Name in"="fill.fraction") -> ("output cluster"=w737:T15)  [unwired: 9 in, 1 out]
          n355 = call "GFG_core.vi"("Variable Name in"="xy.voltage.map") -> ("Variant Out"=w730:variant)  [unwired: 12 in, 6 out]
          n356 = property class="DigNum"(reference=w739, "DisabledEnum"=T4."Enabled" ("Disabled")) -> ()  [unwired: 1 in, 2 out]
          n357 = Unbundle By Name(w737) -> ("DigitalRef"=w738:refnum<vi>)
          n358 = Variant To Data(type=T8 {"xyvoltagefor2frames"=[], "x.pixels"=0.0, "nomin.x.pixels"=0.0, "y.pixels"=0.0, "fill.fraction"=0.0, "x.bidirectional"=FALSE, "y.bidirectional"=FALSE} ("output cluster"), Variant=w730) -> (data=w727:T8, error out=→"error out 3":errorcluster)  [unwired: 1 in]
          n359 = call "GFG_core.vi"("Variable Name in"="experiment type", "Variant in"=T7 "XYT" ("experiment type"), "Action"=enum16{"Init", "Set", "Get"}."Set") -> ()  [unwired: 10 in, 7 out]
          n360 = property class="DigNum"(reference=w738, "DisabledEnum"=T4."Enabled" ("Disabled")) -> ()  [unwired: 1 in, 2 out]
          n361 = call "GFG refresh all variables.vi"("Variables to refresh"=string[] ["pixel resolution", "x.bidirectional"] ("All Variable Names")) -> ()  [unwired: 11 in]
          n362 = call "line scan enable disable.vi"("Page Enabled State"=T9."Page Disabled & Grayed") -> ()  [unwired: 11 in]
          n363 = call "GFG_core.vi"("Variable Name in"="no..of.frames.for.frame.scan", "Action"=enum16{"Init", "Set", "Get"}."Get") -> ("Variable Name Out"=w743:string)  [unwired: 11 in, 6 out]
          n364 = Unbundle(w727) -> ("x.pixels"=w725:dbl, "nomin.x.pixels"=w723:dbl, "y.pixels"=w721:dbl, "fill.fraction"=w719:dbl, "x.bidirectional"=w717:bool, "y.bidirectional"=w715:bool)  [unwired: 1 out]
          n365 = call "GFG_core.vi"("Variable Name in"="y.bidirectional" ("Tag in"), "Variant in"=w715, "Action"=w714) -> ()  [unwired: 10 in, 7 out]
          n366 = call "GFG_core.vi"("Variable Name in"="x.bidirectional" ("Tag in"), "Variant in"=w717, "Action"=w714) -> ()  [unwired: 10 in, 7 out]
          n367 = call "GFG_core.vi"("Variable Name in"="fill.fraction", "Variant in"=w719, "Action"=w714) -> ()  [unwired: 10 in, 7 out]
          n368 = call "GFG_core.vi"("Variable Name in"="nomin.x.pixels", "Variant in"=w723, "Action"=w714) -> ()  [unwired: 10 in, 7 out]
          n369 = call "GFG_core.vi"("Variable Name in"=" no..of.frames.to.acquire", "Variant in"=w743, "Action"=enum16{"Init", "Set", "Get"}."Set") -> ()  [unwired: 10 in, 7 out]
          n370 = call "GFG_core.vi"("Variable Name in"="x.pixels" ("Tag in"), "Variant in"=w725, "Action"=w714) -> ()  [unwired: 10 in, 7 out]
          n371 = call "GFG_core.vi"("Variable Name in"="y.pixels" ("Tag in"), "Variant in"=w721, "Action"=w714) -> ()  [unwired: 10 in, 7 out]
        }
        frame "Z Stack" {
          w750 = enum16{"Init", "Set", "Get"}."Set" ("Action")
          n372 = call "GFG_core.vi"("Variable Name in"="xy.voltage.map") -> ("Variant Out"=w766:variant)  [unwired: 12 in, 6 out]
          n373 = Variant To Data(type=T8 {"xyvoltagefor2frames"=[], "x.pixels"=0.0, "nomin.x.pixels"=0.0, "y.pixels"=0.0, "fill.fraction"=0.0, "x.bidirectional"=FALSE, "y.bidirectional"=FALSE} ("output cluster"), Variant=w766) -> (data=w763:T8, error out=→"error out 4":errorcluster)  [unwired: 1 in]
          n374 = call "control tab sliding.vi"("close(T)/open(F)"=FALSE, "String"="advanced settings slider tab") -> ()  [unwired: 10 in]
          n375 = call "GFG_core.vi"("Variable Name in"="pos  pockels cell PMT Data") -> ("Variant Out"=w773:variant)  [unwired: 12 in, 6 out]
          n376 = call "GFG_core.vi"("Variable Name in"="advanced settings inner tab", "Variant in"=advanced_settings_inner_tab_CTL."Zstack data" ("advanced settings inner tab"), "Action"=enum16{"Init", "Set", "Get"}."Set") -> ()  [unwired: 10 in, 7 out]
          n377 = call "GFG_core.vi"("Variable Name in"="experiment type", "Variant in"=T7 "XYTZ" ("experiment type"), "Action"=enum16{"Init", "Set", "Get"}."Set") -> ()  [unwired: 10 in, 7 out]
          n378 = Unbundle(w763) -> ("x.pixels"=w761:dbl, "nomin.x.pixels"=w759:dbl, "y.pixels"=w757:dbl, "fill.fraction"=w755:dbl, "x.bidirectional"=w753:bool, "y.bidirectional"=w751:bool)  [unwired: 1 out]
          n379 = call "GFG_core.vi"("Variable Name in"="y.bidirectional" ("Tag in"), "Variant in"=w751, "Action"=w750) -> ()  [unwired: 10 in, 7 out]
          n380 = call "GFG_core.vi"("Variable Name in"="x.bidirectional" ("Tag in"), "Variant in"=w753, "Action"=w750) -> ()  [unwired: 10 in, 7 out]
          n381 = call "GFG_core.vi"("Variable Name in"="fill.fraction", "Variant in"=w755, "Action"=w750) -> ()  [unwired: 10 in, 7 out]
          n382 = call "GFG_core.vi"("Variable Name in"="nomin.x.pixels", "Variant in"=w759, "Action"=w750) -> ()  [unwired: 10 in, 7 out]
          n383 = Variant To Data(type=dbl[][] [[0.0, 0.0], [1.0, 0.0]] ("pos  pockels cell PMT Data"), Variant=w773) -> (data=w771:dbl[][])  [unwired: 1 in, 1 out]
          n384 = call "GFG_core.vi"("Variable Name in"="x.pixels" ("Tag in"), "Variant in"=w761, "Action"=w750) -> ()  [unwired: 10 in, 7 out]
          n385 = call "GFG_core.vi"("Variable Name in"="y.pixels" ("Tag in"), "Variant in"=w757, "Action"=w750) -> ()  [unwired: 10 in, 7 out]
          n386 = Empty Array?(array=w771) -> (empty?=w769:bool)
          n387 = Not(x=w769) -> (.not. x?=w768:bool)
          n388 = case shown="True" w768 {
            frame False {
            }
            frame True {
              n389 = call "GFG refresh all variables.vi"("Variables to refresh"=string[] ["frames.per.plane"] ("All Variable Names")) -> ()  [unwired: 11 in]
            }
          }
        }
        frame "2D line scan" {
          n390 = call "GFG_core.vi"("Variable Name in"="experiment type", "Variant in"=T7 "[xy]T" ("experiment type"), "Action"=enum16{"Init", "Set", "Get"}."Set") -> ()  [unwired: 10 in, 7 out]
        }
        frame "piezo" {
          w788 = enum16{"Init", "Set", "Get"}."Set" ("Action")
          n391 = call "GFG_core.vi"("Variable Name in"="xy.voltage.map") -> ("Variant Out"=w804:variant)  [unwired: 12 in, 6 out]
          n392 = Variant To Data(type=T8 {"xyvoltagefor2frames"=[], "x.pixels"=0.0, "nomin.x.pixels"=0.0, "y.pixels"=0.0, "fill.fraction"=0.0, "x.bidirectional"=FALSE, "y.bidirectional"=FALSE} ("output cluster"), Variant=w804) -> (data=w801:T8, error out=→"error out 5":errorcluster)  [unwired: 1 in]
          n393 = Build Array("no.of.cycles.to.scan" ("Variable Name")) -> (w806:string[])
          n394 = call "GFG refresh all variables.vi"("Variables to refresh"=w806) -> ()  [unwired: 11 in]
          n395 = Unbundle(w801) -> ("x.pixels"=w799:dbl, "nomin.x.pixels"=w797:dbl, "y.pixels"=w795:dbl, "fill.fraction"=w793:dbl, "x.bidirectional"=w791:bool, "y.bidirectional"=w789:bool)  [unwired: 1 out]
          n396 = call "GFG_core.vi"("Variable Name in"="y.bidirectional" ("Tag in"), "Variant in"=w789, "Action"=w788) -> ()  [unwired: 10 in, 7 out]
          n397 = call "GFG_core.vi"("Variable Name in"="x.bidirectional" ("Tag in"), "Variant in"=w791, "Action"=w788) -> ()  [unwired: 10 in, 7 out]
          n398 = call "GFG_core.vi"("Variable Name in"="fill.fraction", "Variant in"=w793, "Action"=w788) -> ()  [unwired: 10 in, 7 out]
          n399 = call "GFG_core.vi"("Variable Name in"="nomin.x.pixels", "Variant in"=w797, "Action"=w788) -> ()  [unwired: 10 in, 7 out]
          n400 = call "GFG_core.vi"("Variable Name in"="x.pixels" ("Tag in"), "Variant in"=w799, "Action"=w788) -> ()  [unwired: 10 in, 7 out]
          n401 = call "GFG_core.vi"("Variable Name in"="y.pixels" ("Tag in"), "Variant in"=w795, "Action"=w788) -> ()  [unwired: 10 in, 7 out]
        }
      }
    }
    frame "MAIN.Image.panels." {
      n402 = Variant To Data(type=MAIN_Image_panel_tab_Control_type_def."Channel 1" ("MAIN Image panels"), Variant=w817) -> (data=w816:T11)  [unwired: 1 in, 1 out]
      n403 = call-poly "GFGpolyGet.vi"("Variable Name in"="Histograms tab") -> ("output cluster"=w812:T15)  [unwired: 9 in, 1 out]
      n404 = case shown="\"Channel 2\"" w816 {
        tunnel: w815 -> [w823 w829 w835 w841 w851 w854 w859 w870]
        tunnel: [w823 w829 w835 w841 w851 w854 w859 w870] -> w814
        tunnel: [Histogram_tab."hist Ch 1" ("Histograms tab") Histogram_tab."hist Ch 2" ("Histograms tab") Histogram_tab."hist Ch 3" ("Histograms tab") Histogram_tab."hist Ch 4" ("Histograms tab") Histogram_tab."hist Ch 1" ("Histograms tab") Histogram_tab."hist Ch 1" ("Histograms tab") Histogram_tab."hist Ch 1" ("Histograms tab") Histogram_tab."hist Ch 1" ("Histograms tab")] -> w809
        frame "Channel 1" {
          n405 = call-poly "GFGpolyGet.vi"("Variable Name in"="autocorrect.startdelay") -> ("output cluster"=w819:T15)  [unwired: 9 in, 1 out]
          n406 = Unbundle By Name(w819) -> ("BooleanRef"=w820:refnum<vi>)
          n407 = property class="Bool"(reference=w820, "DisabledEnum"=T4."Enabled" ("Disabled")) -> ()  [unwired: 1 in, 2 out]
        }
        frame "Channel 2" {
          n408 = call-poly "GFGpolyGet.vi"("Variable Name in"="autocorrect.startdelay") -> ("output cluster"=w825:T15)  [unwired: 9 in, 1 out]
          n409 = Unbundle By Name(w825) -> ("BooleanRef"=w826:refnum<vi>)
          n410 = property class="Bool"(reference=w826, "DisabledEnum"=T4."Enabled" ("Disabled")) -> ()  [unwired: 1 in, 2 out]
        }
        frame "Channel 3" {
          n411 = call-poly "GFGpolyGet.vi"("Variable Name in"="autocorrect.startdelay") -> ("output cluster"=w831:T15)  [unwired: 9 in, 1 out]
          n412 = Unbundle By Name(w831) -> ("BooleanRef"=w832:refnum<vi>)
          n413 = property class="Bool"(reference=w832, "DisabledEnum"=T4."Enabled" ("Disabled")) -> ()  [unwired: 1 in, 2 out]
        }
        frame "Channel 4" {
          n414 = call-poly "GFGpolyGet.vi"("Variable Name in"="autocorrect.startdelay") -> ("output cluster"=w837:T15)  [unwired: 9 in, 1 out]
          n415 = Unbundle By Name(w837) -> ("BooleanRef"=w838:refnum<vi>)
          n416 = property class="Bool"(reference=w838, "DisabledEnum"=T4."Enabled" ("Disabled")) -> ()  [unwired: 1 in, 2 out]
        }
        frame "all channels" {
          n417 = call-poly "GFGpolyGet.vi"() -> ("DisplayRefsOut(generic class)"=w850:T14)  [unwired: 10 in, 1 out]
          n418 = call-poly "GFGpolyGet.vi"() -> ("Image Refs Out"=w849:T17)  [unwired: 10 in, 1 out]
          n419 = Cluster To Array(cluster=w850) -> (array=w848:refnum<vi>[])
          n420 = Cluster To Array(cluster=w849) -> (array=w847:T16[])
          n421 = call "set initial zoom.vi"("reset?"=TRUE, "Image Refs In"=w847, "DisplayRefsIn(generic class)"=w848) -> ()  [unwired: 9 in]
          n422 = call-poly "GFGpolyGet.vi"("Variable Name in"="autocorrect.startdelay") -> ("output cluster"=w843:T15)  [unwired: 9 in, 1 out]
          n423 = Unbundle By Name(w843) -> ("BooleanRef"=w844:refnum<vi>)
          n424 = property class="Bool"(reference=w844, "DisabledEnum"=T4."Disabled and Grayed Out" ("Disabled")) -> ()  [unwired: 1 in, 2 out]
        }
        frame "RGB overlay" {
          n425 = call-poly "GFGpolyGet.vi"("Variable Name in"="autocorrect.startdelay") -> ("output cluster"=w856:T15)  [unwired: 9 in, 1 out]
          n426 = Unbundle By Name(w856) -> ("BooleanRef"=w857:refnum<vi>)
          n427 = property class="Bool"(reference=w857, "DisabledEnum"=T4."Disabled and Grayed Out" ("Disabled")) -> ()  [unwired: 1 in, 2 out]
        }
        frame "ROI" {
          n428 = call-poly "GFGpolyGet.vi"("Variable Name in"="autocorrect.startdelay") -> ("output cluster"=w863:T15)  [unwired: 9 in, 1 out]
          n429 = Unbundle By Name(w863) -> ("BooleanRef"=w862:refnum<vi>)
          n430 = property class="Bool"(reference=w862, "DisabledEnum"=T4."Enabled" ("Disabled")) -> ()  [unwired: 1 in, 2 out]
        }
        frame "arbitrary line scan" {
          n431 = call-poly "GFGpolyGet.vi"("Variable Name in"="autocorrect.startdelay") -> ("output cluster"=w867:T15)  [unwired: 9 in, 1 out]
          n432 = Unbundle By Name(w867) -> ("BooleanRef"=w868:refnum<vi>)
          n433 = property class="Bool"(reference=w868, "DisabledEnum"=T4."Disabled and Grayed Out" ("Disabled")) -> ()  [unwired: 1 in, 2 out]
        }
      }
      n434 = Unbundle By Name(w812) -> ("TabControlRef"=w810:refnum<vi>)
      n435 = property class="TabCtl"(reference=w810, "Value"=w809) -> ()  [unwired: 1 in, 2 out]
    }
    frame "piezo.active" {
      n436 = call-poly "GFGpolyGet.vi"("Variable Name in"="Laser.Power") -> ("output cluster"=w878:T15)  [unwired: 9 in, 1 out]
      n437 = Unbundle By Name(w878) -> ("KnobRef"=w877:refnum<vi>)
      n438 = Variant To Data(type=TRUE, Variant=w872) -> (data=w873:bool)  [unwired: 1 in, 1 out]
      n439 = Select(t=T4."Disabled and Grayed Out" ("Disabled"), s=w873, f=T4."Enabled" ("Disabled")) -> (s? t:f=w874:T4)
      n440 = property class="Knob"(reference=w877, "DisabledEnum"=w874) -> ()  [unwired: 1 in, 2 out]
    }
    frame "Objective" {
      n441 = Variant To Data(type=u16 0, Variant=w899) -> (data=w881:u16)  [unwired: 1 in, 1 out]
      n442 = Increment(x=w881) -> (x+1=w893:u16)
      n443 = Number To Decimal String(number=w893) -> (decimal integer string=w886:string)  [unwired: 1 in]
      n444 = call "GFG_core.vi"("Variable Name in"="active.objective", "Variant in"=w881, "Action"=enum16{"Init", "Set", "Get"}."Set") -> ()  [unwired: 10 in, 7 out]
      n445 = Concatenate Strings("obj", w886, ".max.field.of.view") -> (w894:string)
      n446 = Concatenate Strings("obj", w886, ".voltage.for.max.field.of.view") -> (w887:string)
      n447 = call-poly "GFGpolyGet.vi"("Variable Name in"=w894) -> ("Numeric"=w891:dbl)  [unwired: 8 in, 2 out]
      n448 = call-poly "GFGpolyGet.vi"("Variable Name in"=w887) -> ("Numeric"=w884:dbl)  [unwired: 8 in, 2 out]
      n449 = call "GFG_core.vi"("Variable Name in"="max.field.of.view", "Variant in"=w891, "Action"=enum16{"Init", "Set", "Get"}."Set") -> ()  [unwired: 10 in, 7 out]
      n450 = call "GFG_core.vi"("Variable Name in"="voltage.for.max.field.of.view", "Variant in"=w884, "Action"=enum16{"Init", "Set", "Get"}."Set") -> ()  [unwired: 10 in, 7 out]
    }
    frame "shutdown" {
      w901 = enum16{"Init", "Set", "Get"}."Set" ("Action")
      n451 = call "GFG_core.vi"("Variable Name in"="xy.voltage.map") -> ("Variant Out"=w917:variant)  [unwired: 12 in, 6 out]
      n452 = Variant To Data(type=T8 {"xyvoltagefor2frames"=[], "x.pixels"=0.0, "nomin.x.pixels"=0.0, "y.pixels"=0.0, "fill.fraction"=0.0, "x.bidirectional"=FALSE, "y.bidirectional"=FALSE} ("output cluster"), Variant=w917) -> (data=w914:T8, error out=→"error out 6":errorcluster)  [unwired: 1 in]
      n453 = Unbundle(w914) -> ("x.pixels"=w912:dbl, "nomin.x.pixels"=w910:dbl, "y.pixels"=w908:dbl, "fill.fraction"=w906:dbl, "x.bidirectional"=w904:bool, "y.bidirectional"=w902:bool)  [unwired: 1 out]
      n454 = call "GFG_core.vi"("Variable Name in"="fill.fraction", "Variant in"=w906, "Action"=w901) -> ()  [unwired: 10 in, 7 out]
      n455 = call "GFG_core.vi"("Variable Name in"="nomin.x.pixels", "Variant in"=w910, "Action"=w901) -> ()  [unwired: 10 in, 7 out]
      n456 = call "GFG_core.vi"("Variable Name in"="y.pixels" ("Tag in"), "Variant in"=w908, "Action"=w901) -> ()  [unwired: 10 in, 7 out]
      n457 = call "GFG_core.vi"("Variable Name in"="x.pixels" ("Tag in"), "Variant in"=w912, "Action"=w901) -> ()  [unwired: 10 in, 7 out]
      n458 = call "GFG_core.vi"("Variable Name in"="y.bidirectional" ("Tag in"), "Variant in"=w902, "Action"=w901) -> ()  [unwired: 10 in, 7 out]
      n459 = call "GFG_core.vi"("Variable Name in"="x.bidirectional" ("Tag in"), "Variant in"=w904, "Action"=w901) -> ()  [unwired: 10 in, 7 out]
    }
    frame "trigger.enum" {
      w939 = "Initial delay\n[frames]"
      w940 = "Pulse\nevery n frames"
      n460 = Build Array("Pulse\nfrequency [Hz]", "Initial delay\n[ms]") -> (w946:string[])
      n461 = Build Array(w940, w939) -> (w947:string[])
      n462 = Build Array("Pulse\nevery n frames", "Pulse\nfrequency [Hz]") -> (w924:string[])
      n463 = call-poly "GFGpolyGet.vi"("Variable Name in"="pulse.Boolean") -> ("Boolean Value OUT"=w941:bool)  [unwired: 9 in, 1 out]
      n464 = call-poly "GFGpolyGet.vi"("Variable Name in"="pulse.Boolean") -> ("output cluster"=w937:T15)  [unwired: 9 in, 1 out]
      n465 = for {
        tunnel: w947 -> [w969] mode=indexing
        tunnel: w941 -> [w966]
        n466 = call-poly "GFGpolyGet.vi"("Variable Name in"=w969) -> ("output cluster"=w968:T15)  [unwired: 9 in, 1 out]
        n467 = Unbundle By Name(w968) -> ("DigitalRef"=w967:refnum<vi>)
        n468 = property class="DigNum"(reference=w967, "Visible"=w966) -> ()  [unwired: 1 in, 2 out]
      }
      n469 = Build Array("Initial delay [ms]", "Pulse duration [ms]", "Pulse frequency [Hz]", w940, w939) -> (w954:string[])
      n470 = Not(x=w941) -> (.not. x?=w943:bool)
      n471 = for {
        tunnel: w946 -> [w965] mode=indexing
        tunnel: w943 -> [w962]
        n472 = call-poly "GFGpolyGet.vi"("Variable Name in"=w965) -> ("output cluster"=w964:T15)  [unwired: 9 in, 1 out]
        n473 = Unbundle By Name(w964) -> ("DigitalRef"=w963:refnum<vi>)
        n474 = property class="DigNum"(reference=w963, "Visible"=w962) -> ()  [unwired: 1 in, 2 out]
      }
      n475 = Variant To Data(type=trigger_enum."legacy frame pulser PFI4" ("trigger.enum"), Variant=w953) -> (data=w930:T13)  [unwired: 1 in, 1 out]
      n476 = Equal?(x=w930, y=trigger_enum."legacy frame pulser PFI4" ("trigger.enum")) -> (x = y?=w951:bool)
      n477 = Equal?(x=w930, y=trigger_enum."trigger off" ("trigger.enum")) -> (x = y?=w931:bool)
      n478 = Not Equal?(x=w930, y=trigger_enum."continuous pulses" ("trigger.enum")) -> (x != y?=w925:bool)
      n479 = Select(t=T4."Disabled and Grayed Out" ("Disabled"), s=w925, f=T4."Enabled" ("Disabled")) -> (s? t:f=w926:T4)
      n480 = Or(x=w951, y=w931) -> (x .or. y?=w933:bool)
      n481 = Unbundle By Name(w937) -> ("BooleanRef"=w938:refnum<vi>)
      n482 = Select(t=T4."Disabled and Grayed Out" ("Disabled"), s=w933, f=T4."Enabled" ("Disabled")) -> (s? t:f=w935:T4)
      n483 = property class="Bool"(reference=w938, "DisabledEnum"=w935) -> ()  [unwired: 1 in, 2 out]
      n484 = for {
        tunnel: w954 -> [w974] mode=indexing
        tunnel: w935 -> [w971]
        tunnel: [w970] -> w921 mode=indexing
        n485 = call-poly "GFGpolyGet.vi"("Variable Name in"=w974) -> ("output cluster"=w973:T15)  [unwired: 9 in, 1 out]
        n486 = Unbundle By Name(w973) -> ("DigitalRef"=w972:refnum<vi>)
        n487 = property class="DigNum"(reference=w972, "DisabledEnum"=w971) -> (error out=w970:errorcluster)  [unwired: 1 in, 1 out]
      }
      n488 = for {
        tunnel: w924 -> [w961] mode=indexing
        tunnel: w926 -> [w958]
        tunnel: w921 -> [_] mode=indexing
        n489 = call-poly "GFGpolyGet.vi"("Variable Name in"=w961) -> ("output cluster"=w960:T15)  [unwired: 9 in, 1 out]
        n490 = Unbundle By Name(w960) -> ("DigitalRef"=w959:refnum<vi>)
        n491 = property class="DigNum"(reference=w959, "DisabledEnum"=w958) -> ()  [unwired: 1 in, 2 out]
      }
    }
    frame "pulse.Boolean" {
      n492 = Variant To Data(type=TRUE, Variant=w981) -> (data=w977:bool)  [unwired: 1 in, 1 out]
      n493 = Build Array("Pulse\nevery n frames", "Initial delay\n[frames]") -> (w983:string[])
      n494 = Build Array("Pulse\nfrequency [Hz]", "Initial delay\n[ms]") -> (w980:string[])
      n495 = Not(x=w977) -> (.not. x?=w976:bool)
      n496 = for {
        tunnel: w983 -> [w993] mode=indexing
        tunnel: w977 -> [w990]
        n497 = call-poly "GFGpolyGet.vi"("Variable Name in"=w993) -> ("output cluster"=w992:T15)  [unwired: 9 in, 1 out]
        n498 = Unbundle By Name(w992) -> ("DigitalRef"=w991:refnum<vi>)
        n499 = property class="DigNum"(reference=w991, "Visible"=w990) -> ()  [unwired: 1 in, 2 out]
      }
      n500 = for {
        tunnel: w980 -> [w989] mode=indexing
        tunnel: w976 -> [w986]
        n501 = call-poly "GFGpolyGet.vi"("Variable Name in"=w989) -> ("output cluster"=w988:T15)  [unwired: 9 in, 1 out]
        n502 = Unbundle By Name(w988) -> ("DigitalRef"=w987:refnum<vi>)
        n503 = property class="DigNum"(reference=w987, "Visible"=w986) -> ()  [unwired: 1 in, 2 out]
      }
    }
  }
  "Timeout OUT" <- w2
  "shutdown?" <- w1
